vi "函数类型3测试.vi"() -> ()   [LabVIEW 2010]
panel:
  in  "加载配置文件":u16(ring) items=["123.xls", "12333.xls", "1234.xls", "12345.xls", "123666.xls", "12368966.xls"]
  in  "是否取反":bool
  in  "保持输出":bool
  in  "同步_A2":i32
  in  "同步_A1":i32
  in  "数组_输入值":enum16{"0", "1"}[][](array[ring])
  in  "数组_选择?":bool[][](array[boolean])
  in  "btn_置1_5":bool
  in  "btn_置1_4":bool
  in  "btn_置1_3":bool
  in  "btn_置1_2":bool
  in  "btn_全选_5":bool
  in  "btn_全选_4":bool
  in  "btn_全选_3":bool
  in  "btn_全选_2":bool
  in  "btn_置1_1":bool
  in  "btn_全选_1":bool
  in  "CAN端口":u16
  out "light_80":bool
  out "light_79":bool
  out "light_78":bool
  out "light_77":bool
  out "light_76":bool
  out "light_75":bool
  out "light_74":bool
  out "light_73":bool
  out "light_72":bool
  out "light_71":bool
  out "light_70":bool
  out "light_69":bool
  out "light_68":bool
  out "light_67":bool
  out "light_66":bool
  out "light_65":bool
  in  "输入值_73":enum16{"0", "1"}(ring)
  in  "输入值_80":enum16{"0", "1"}(ring)
  in  "输入值_79":enum16{"0", "1"}(ring)
  in  "输入值_78":enum16{"0", "1"}(ring)
  in  "输入值_77":enum16{"0", "1"}(ring)
  in  "输入值_76":enum16{"0", "1"}(ring)
  in  "输入值_75":enum16{"0", "1"}(ring)
  in  "输入值_74":enum16{"0", "1"}(ring)
  in  "输入值_65":enum16{"0", "1"}(ring)
  in  "输入值_72":enum16{"0", "1"}(ring)
  in  "输入值_71":enum16{"0", "1"}(ring)
  in  "输入值_70":enum16{"0", "1"}(ring)
  in  "输入值_69":enum16{"0", "1"}(ring)
  in  "输入值_68":enum16{"0", "1"}(ring)
  in  "输入值_67":enum16{"0", "1"}(ring)
  in  "输入值_66":enum16{"0", "1"}(ring)
  in  "单选_第73路":bool
  in  "单选_第80路":bool
  in  "单选_第79路":bool
  in  "单选_第78路":bool
  in  "单选_第77路":bool
  in  "单选_第76路":bool
  in  "单选_第75路":bool
  in  "单选_第74路":bool
  in  "单选_第65路":bool
  in  "单选_第72路":bool
  in  "单选_第71路":bool
  in  "单选_第70路":bool
  in  "单选_第69路":bool
  in  "单选_第68路":bool
  in  "单选_第67路":bool
  in  "单选_第66路":bool
  out "light_64":bool
  out "light_63":bool
  out "light_62":bool
  out "light_61":bool
  out "light_60":bool
  out "light_59":bool
  out "light_58":bool
  out "light_57":bool
  out "light_56":bool
  out "light_55":bool
  out "light_54":bool
  out "light_53":bool
  out "light_52":bool
  out "light_51":bool
  out "light_50":bool
  out "light_49":bool
  in  "输入值_57":enum16{"0", "1"}(ring)
  in  "输入值_64":enum16{"0", "1"}(ring)
  in  "输入值_63":enum16{"0", "1"}(ring)
  in  "输入值_62":enum16{"0", "1"}(ring)
  in  "输入值_61":enum16{"0", "1"}(ring)
  in  "输入值_60":enum16{"0", "1"}(ring)
  in  "输入值_59":enum16{"0", "1"}(ring)
  in  "输入值_58":enum16{"0", "1"}(ring)
  in  "输入值_49":enum16{"0", "1"}(ring)
  in  "输入值_56":enum16{"0", "1"}(ring)
  in  "输入值_55":enum16{"0", "1"}(ring)
  in  "输入值_54":enum16{"0", "1"}(ring)
  in  "输入值_53":enum16{"0", "1"}(ring)
  in  "输入值_52":enum16{"0", "1"}(ring)
  in  "输入值_51":enum16{"0", "1"}(ring)
  in  "输入值_50":enum16{"0", "1"}(ring)
  in  "单选_第57路":bool
  in  "单选_第64路":bool
  in  "单选_第63路":bool
  in  "单选_第62路":bool
  in  "单选_第61路":bool
  in  "单选_第60路":bool
  in  "单选_第59路":bool
  in  "单选_第58路":bool
  in  "单选_第49路":bool
  in  "单选_第56路":bool
  in  "单选_第55路":bool
  in  "单选_第54路":bool
  in  "单选_第53路":bool
  in  "单选_第52路":bool
  in  "单选_第51路":bool
  in  "单选_第50路":bool
  out "light_48":bool
  out "light_47":bool
  out "light_46":bool
  out "light_45":bool
  out "light_44":bool
  out "light_43":bool
  out "light_42":bool
  out "light_41":bool
  out "light_40":bool
  out "light_39":bool
  out "light_38":bool
  out "light_37":bool
  out "light_36":bool
  out "light_35":bool
  out "light_34":bool
  out "light_33":bool
  in  "输入值_41":enum16{"0", "1"}(ring)
  in  "输入值_48":enum16{"0", "1"}(ring)
  in  "输入值_47":enum16{"0", "1"}(ring)
  in  "输入值_46":enum16{"0", "1"}(ring)
  in  "输入值_45":enum16{"0", "1"}(ring)
  in  "输入值_44":enum16{"0", "1"}(ring)
  in  "输入值_43":enum16{"0", "1"}(ring)
  in  "输入值_42":enum16{"0", "1"}(ring)
  in  "输入值_33":enum16{"0", "1"}(ring)
  in  "输入值_40":enum16{"0", "1"}(ring)
  in  "输入值_39":enum16{"0", "1"}(ring)
  in  "输入值_38":enum16{"0", "1"}(ring)
  in  "输入值_37":enum16{"0", "1"}(ring)
  in  "输入值_36":enum16{"0", "1"}(ring)
  in  "输入值_35":enum16{"0", "1"}(ring)
  in  "输入值_34":enum16{"0", "1"}(ring)
  in  "单选_第41路":bool
  in  "单选_第48路":bool
  in  "单选_第47路":bool
  in  "单选_第46路":bool
  in  "单选_第45路":bool
  in  "单选_第44路":bool
  in  "单选_第43路":bool
  in  "单选_第42路":bool
  in  "单选_第33路":bool
  in  "单选_第40路":bool
  in  "单选_第39路":bool
  in  "单选_第38路":bool
  in  "单选_第37路":bool
  in  "单选_第36路":bool
  in  "单选_第35路":bool
  in  "单选_第34路":bool
  out "light_32":bool
  out "light_31":bool
  out "light_30":bool
  out "light_29":bool
  out "light_28":bool
  out "light_27":bool
  out "light_26":bool
  out "light_25":bool
  out "light_24":bool
  out "light_23":bool
  out "light_22":bool
  out "light_21":bool
  out "light_20":bool
  out "light_19":bool
  out "light_18":bool
  out "light_17":bool
  in  "输入值_25":enum16{"0", "1"}(ring)
  in  "输入值_32":enum16{"0", "1"}(ring)
  in  "输入值_31":enum16{"0", "1"}(ring)
  in  "输入值_30":enum16{"0", "1"}(ring)
  in  "输入值_29":enum16{"0", "1"}(ring)
  in  "输入值_28":enum16{"0", "1"}(ring)
  in  "输入值_27":enum16{"0", "1"}(ring)
  in  "输入值_26":enum16{"0", "1"}(ring)
  in  "输入值_17":enum16{"0", "1"}(ring)
  in  "输入值_24":enum16{"0", "1"}(ring)
  in  "输入值_23":enum16{"0", "1"}(ring)
  in  "输入值_22":enum16{"0", "1"}(ring)
  in  "输入值_21":enum16{"0", "1"}(ring)
  in  "输入值_20":enum16{"0", "1"}(ring)
  in  "输入值_19":enum16{"0", "1"}(ring)
  in  "输入值_18":enum16{"0", "1"}(ring)
  in  "单选_第25路":bool
  in  "单选_第32路":bool
  in  "单选_第31路":bool
  in  "单选_第30路":bool
  in  "单选_第29路":bool
  in  "单选_第28路":bool
  in  "单选_第27路":bool
  in  "单选_第26路":bool
  in  "单选_第17路":bool
  in  "单选_第24路":bool
  in  "单选_第23路":bool
  in  "单选_第22路":bool
  in  "单选_第21路":bool
  in  "单选_第20路":bool
  in  "单选_第19路":bool
  in  "单选_第18路":bool
  in  "D_IN_5":string[][](table) caption="表格"
  in  "D_IN_4":string[][](table) caption="表格"
  in  "D_IN_3":string[][](table) caption="表格"
  in  "D_IN_2":string[][](table) caption="表格"
  out "light_16":bool
  out "light_15":bool
  out "light_14":bool
  out "light_13":bool
  out "light_12":bool
  out "light_11":bool
  out "light_10":bool
  out "light_9":bool
  out "light_8":bool
  out "light_7":bool
  out "light_6":bool
  out "light_5":bool
  out "light_4":bool
  out "light_3":bool
  out "light_2":bool
  out "light_1":bool
  in  "输入值_9":enum16{"0", "1"}(ring)
  in  "输入值_16":enum16{"0", "1"}(ring)
  in  "输入值_15":enum16{"0", "1"}(ring)
  in  "输入值_14":enum16{"0", "1"}(ring)
  in  "输入值_13":enum16{"0", "1"}(ring)
  in  "输入值_12":enum16{"0", "1"}(ring)
  in  "输入值_11":enum16{"0", "1"}(ring)
  in  "输入值_10":enum16{"0", "1"}(ring)
  in  "输入值_1":enum16{"0", "1"}(ring)
  in  "输入值_8":enum16{"0", "1"}(ring)
  in  "输入值_7":enum16{"0", "1"}(ring)
  in  "输入值_6":enum16{"0", "1"}(ring)
  in  "输入值_5":enum16{"0", "1"}(ring)
  in  "输入值_4":enum16{"0", "1"}(ring)
  in  "输入值_3":enum16{"0", "1"}(ring)
  in  "输入值_2":enum16{"0", "1"}(ring)
  in  "单选_第9路":bool
  in  "单选_第16路":bool
  in  "单选_第15路":bool
  in  "单选_第14路":bool
  in  "单选_第13路":bool
  in  "单选_第12路":bool
  in  "单选_第11路":bool
  in  "单选_第10路":bool
  in  "单选_第1路":bool
  in  "单选_第8路":bool
  in  "单选_第7路":bool
  in  "单选_第6路":bool
  in  "单选_第5路":bool
  in  "单选_第4路":bool
  in  "单选_第3路":bool
  in  "单选_第2路":bool
  in  "D_IN_1":string[][](table) caption="表格"
  out "关闭？":bool
  out "测试结论":string
  in  "btn_置0":bool
  in  "btn_置1":bool
  in  "btn_反选":bool
  in  "btn_全选":bool
  in  "btn_关闭":bool
  in  "btn_开始试验":bool
  # "第一组数字量测试"
  # "第二组数字量测试"
  # "第三组数字量测试"
  # "第四组数字量测试"
  # "第五组数字量测试"
  # "加载配置文件："
  # "测试结论："
  # "5X16"
  # "5X16"
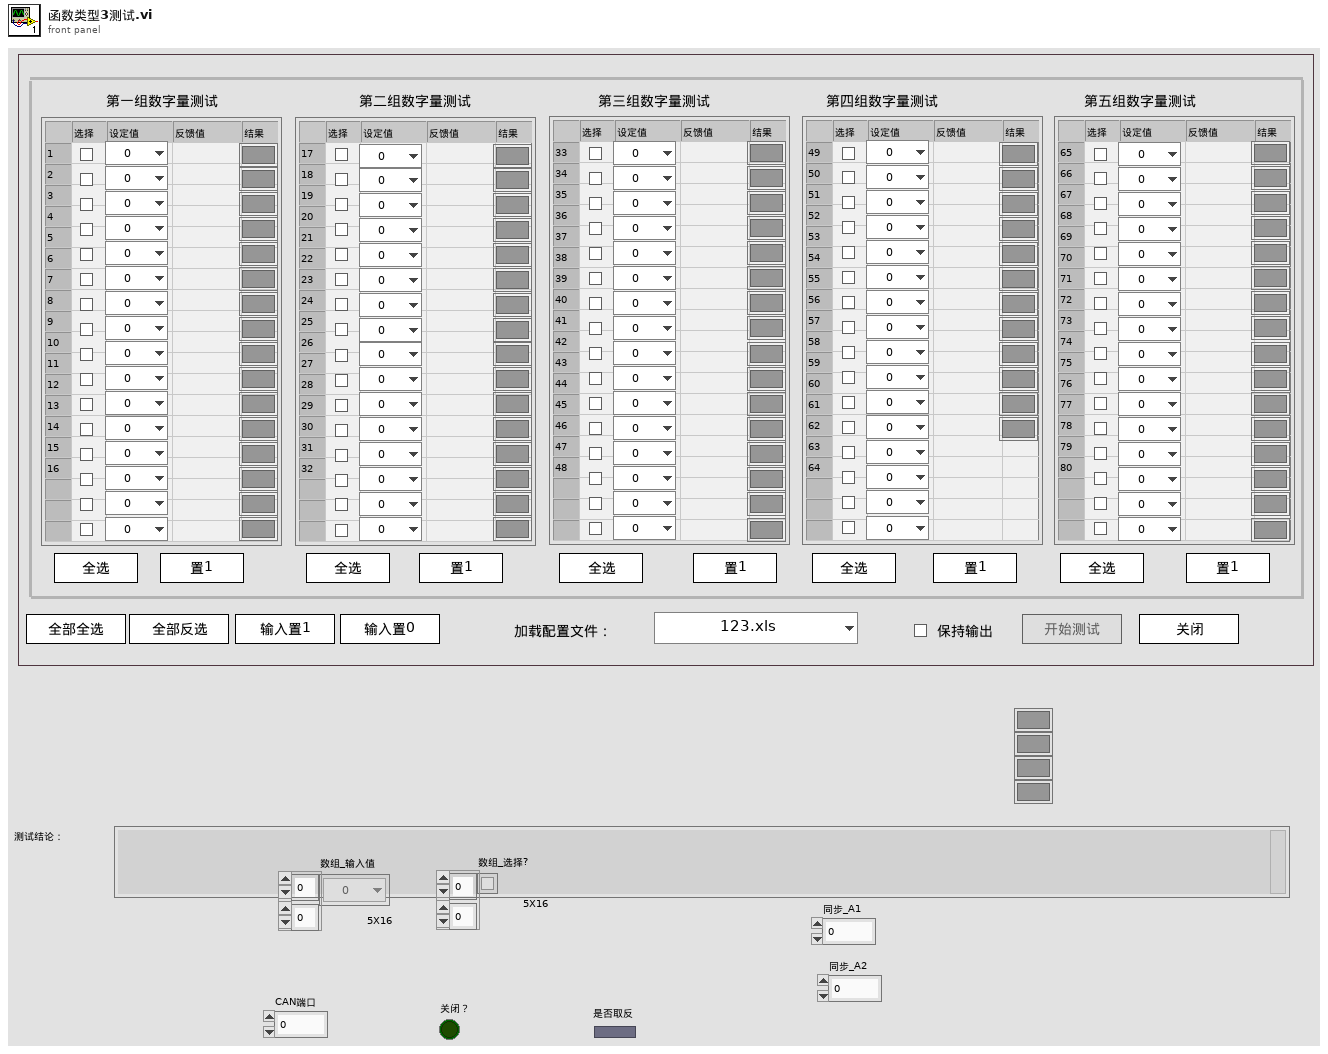
[diagram p1: front panel]
types:
  T1 = enum8{"Enabled", "Disabled", "Disabled and Grayed Out"}
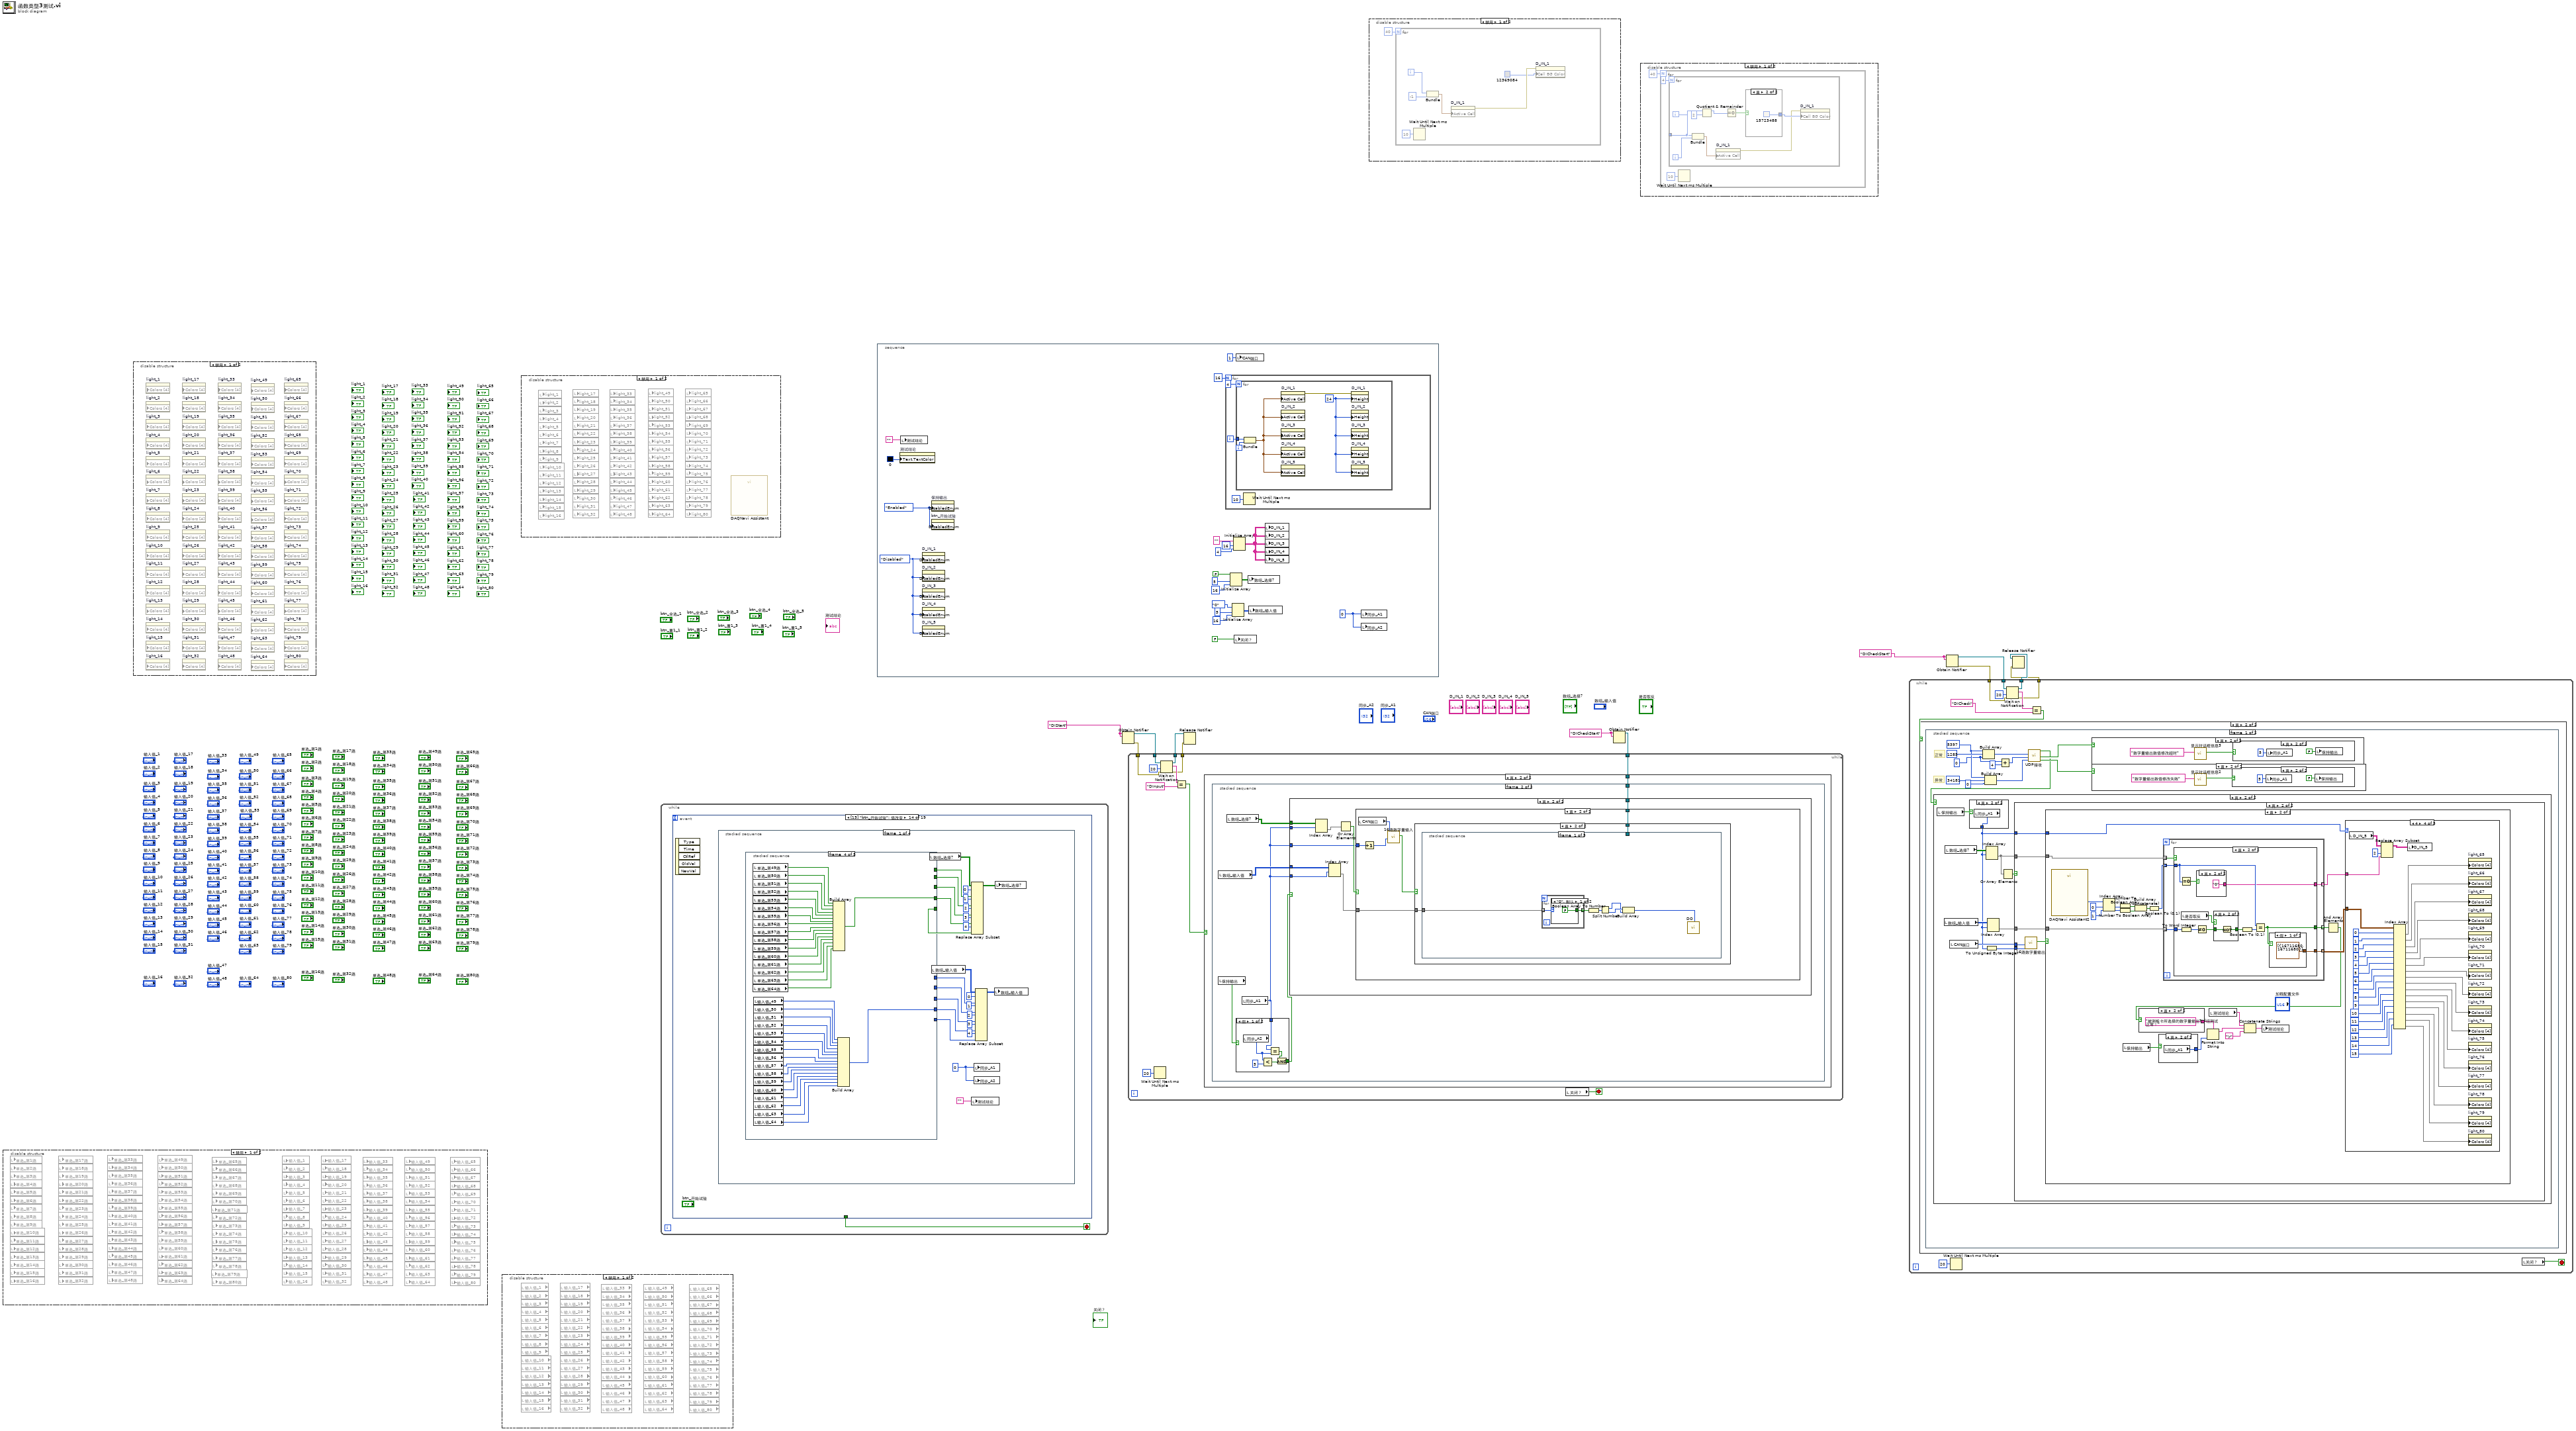
[diagram p0: block diagram]
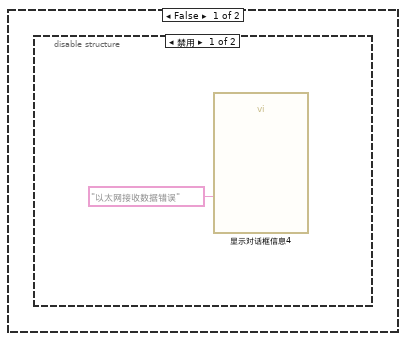
[diagram p7: hidden frame]
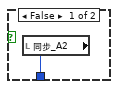
[diagram p9: hidden frame]
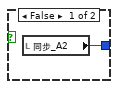
[diagram p12: hidden frame]
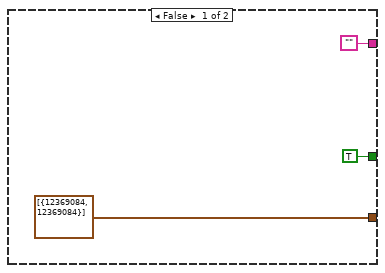
[diagram p13: hidden frame]
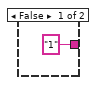
[diagram p15: hidden frame]
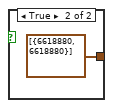
[diagram p16: hidden frame]
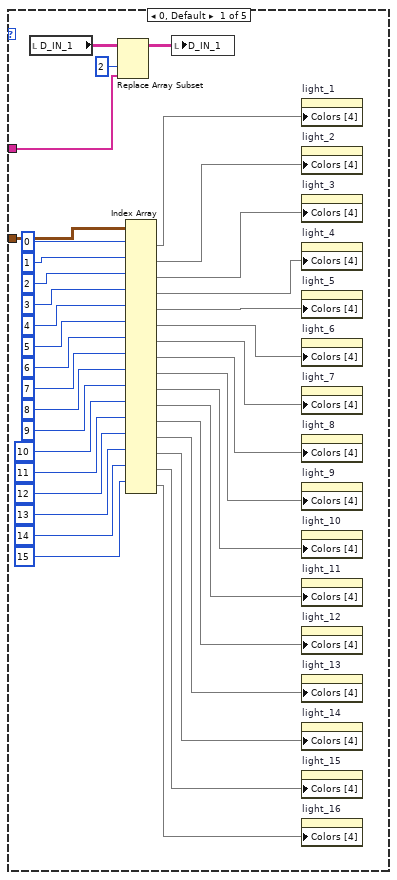
[diagram p17: hidden frame]
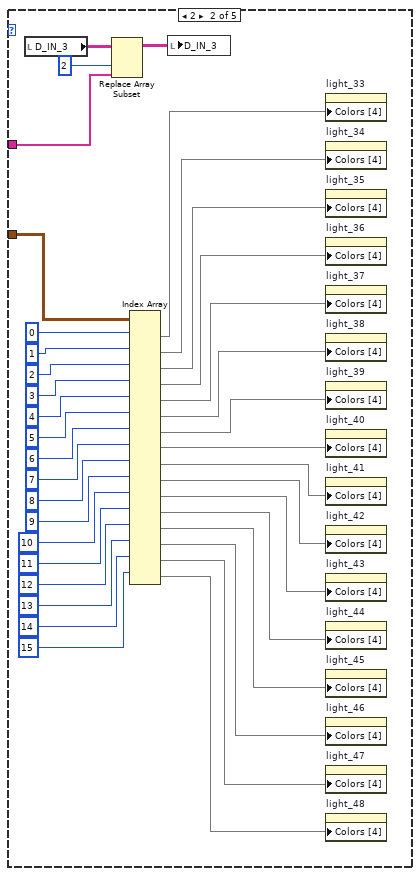
[diagram p18: hidden frame]
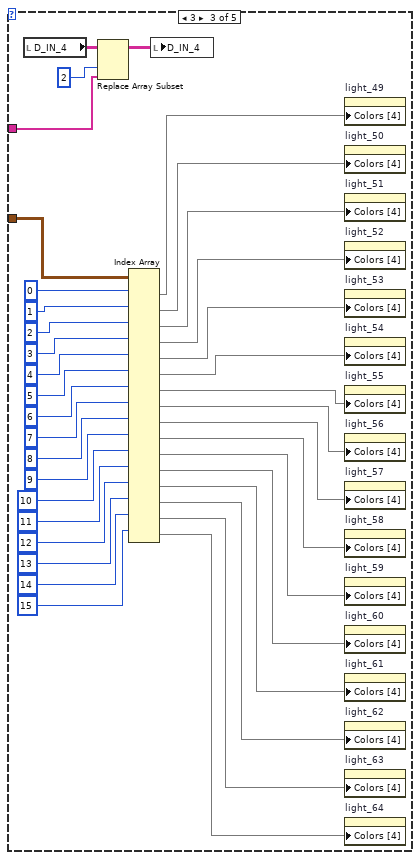
[diagram p19: hidden frame]
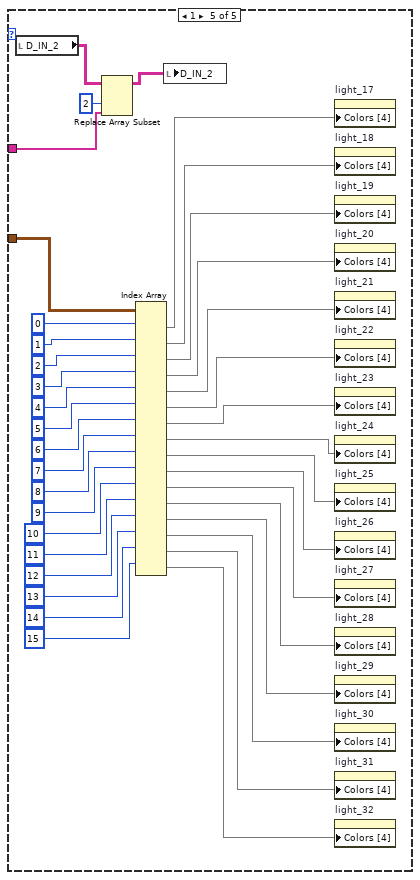
[diagram p20: hidden frame]
diagram:
  w1 = "DICheckStart" ("名称（未命名）")
  w3 = "DICheckStart" ("名称（未命名）")
  w4 = "DIStart" ("名称（未命名）")
  n1 = disable-structure shown="禁用" {
    frame Disabled {
      n2 = local read "单选_第1路"() -> ()  [unwired: 1 in]
      n3 = local read "单选_第2路"() -> ()  [unwired: 1 in]
      n4 = local read "单选_第3路"() -> ()  [unwired: 1 in]
      n5 = local read "单选_第4路"() -> ()  [unwired: 1 in]
      n6 = local read "单选_第5路"() -> ()  [unwired: 1 in]
      n7 = local read "单选_第6路"() -> ()  [unwired: 1 in]
      n8 = local read "单选_第7路"() -> ()  [unwired: 1 in]
      n9 = local read "单选_第8路"() -> ()  [unwired: 1 in]
      n10 = local read "单选_第9路"() -> ()  [unwired: 1 in]
      n11 = local read "单选_第10路"() -> ()  [unwired: 1 in]
      n12 = local read "单选_第11路"() -> ()  [unwired: 1 in]
      n13 = local read "单选_第12路"() -> ()  [unwired: 1 in]
      n14 = local read "单选_第13路"() -> ()  [unwired: 1 in]
      n15 = local read "单选_第14路"() -> ()  [unwired: 1 in]
      n16 = local read "单选_第15路"() -> ()  [unwired: 1 in]
      n17 = local read "单选_第16路"() -> ()  [unwired: 1 in]
      n18 = local read "单选_第17路"() -> ()  [unwired: 1 in]
      n19 = local read "单选_第18路"() -> ()  [unwired: 1 in]
      n20 = local read "单选_第19路"() -> ()  [unwired: 1 in]
      n21 = local read "单选_第20路"() -> ()  [unwired: 1 in]
      n22 = local read "单选_第21路"() -> ()  [unwired: 1 in]
      n23 = local read "单选_第22路"() -> ()  [unwired: 1 in]
      n24 = local read "单选_第23路"() -> ()  [unwired: 1 in]
      n25 = local read "单选_第24路"() -> ()  [unwired: 1 in]
      n26 = local read "单选_第25路"() -> ()  [unwired: 1 in]
      n27 = local read "单选_第26路"() -> ()  [unwired: 1 in]
      n28 = local read "单选_第27路"() -> ()  [unwired: 1 in]
      n29 = local read "单选_第28路"() -> ()  [unwired: 1 in]
      n30 = local read "单选_第29路"() -> ()  [unwired: 1 in]
      n31 = local read "单选_第30路"() -> ()  [unwired: 1 in]
      n32 = local read "单选_第31路"() -> ()  [unwired: 1 in]
      n33 = local read "单选_第32路"() -> ()  [unwired: 1 in]
      n34 = local read "单选_第33路"() -> ()  [unwired: 1 in]
      n35 = local read "单选_第34路"() -> ()  [unwired: 1 in]
      n36 = local read "单选_第35路"() -> ()  [unwired: 1 in]
      n37 = local read "单选_第36路"() -> ()  [unwired: 1 in]
      n38 = local read "单选_第37路"() -> ()  [unwired: 1 in]
      n39 = local read "单选_第38路"() -> ()  [unwired: 1 in]
      n40 = local read "单选_第39路"() -> ()  [unwired: 1 in]
      n41 = local read "单选_第40路"() -> ()  [unwired: 1 in]
      n42 = local read "单选_第41路"() -> ()  [unwired: 1 in]
      n43 = local read "单选_第42路"() -> ()  [unwired: 1 in]
      n44 = local read "单选_第43路"() -> ()  [unwired: 1 in]
      n45 = local read "单选_第44路"() -> ()  [unwired: 1 in]
      n46 = local read "单选_第45路"() -> ()  [unwired: 1 in]
      n47 = local read "单选_第46路"() -> ()  [unwired: 1 in]
      n48 = local read "单选_第47路"() -> ()  [unwired: 1 in]
      n49 = local read "单选_第48路"() -> ()  [unwired: 1 in]
      n50 = local read "单选_第49路"() -> ()  [unwired: 1 in]
      n51 = local read "单选_第50路"() -> ()  [unwired: 1 in]
      n52 = local read "单选_第51路"() -> ()  [unwired: 1 in]
      n53 = local read "单选_第52路"() -> ()  [unwired: 1 in]
      n54 = local read "单选_第53路"() -> ()  [unwired: 1 in]
      n55 = local read "单选_第54路"() -> ()  [unwired: 1 in]
      n56 = local read "单选_第55路"() -> ()  [unwired: 1 in]
      n57 = local read "单选_第56路"() -> ()  [unwired: 1 in]
      n58 = local read "单选_第57路"() -> ()  [unwired: 1 in]
      n59 = local read "单选_第58路"() -> ()  [unwired: 1 in]
      n60 = local read "单选_第59路"() -> ()  [unwired: 1 in]
      n61 = local read "单选_第60路"() -> ()  [unwired: 1 in]
      n62 = local read "单选_第61路"() -> ()  [unwired: 1 in]
      n63 = local read "单选_第62路"() -> ()  [unwired: 1 in]
      n64 = local read "单选_第63路"() -> ()  [unwired: 1 in]
      n65 = local read "单选_第64路"() -> ()  [unwired: 1 in]
      n66 = local read "单选_第71路"() -> ()  [unwired: 1 in]
      n67 = local read "单选_第79路"() -> ()  [unwired: 1 in]
      n68 = local read "单选_第65路"() -> ()  [unwired: 1 in]
      n69 = local read "单选_第66路"() -> ()  [unwired: 1 in]
      n70 = local read "单选_第67路"() -> ()  [unwired: 1 in]
      n71 = local read "单选_第68路"() -> ()  [unwired: 1 in]
      n72 = local read "单选_第69路"() -> ()  [unwired: 1 in]
      n73 = local read "单选_第70路"() -> ()  [unwired: 1 in]
      n74 = local read "单选_第72路"() -> ()  [unwired: 1 in]
      n75 = local read "单选_第73路"() -> ()  [unwired: 1 in]
      n76 = local read "单选_第74路"() -> ()  [unwired: 1 in]
      n77 = local read "单选_第75路"() -> ()  [unwired: 1 in]
      n78 = local read "单选_第76路"() -> ()  [unwired: 1 in]
      n79 = local read "单选_第77路"() -> ()  [unwired: 1 in]
      n80 = local read "单选_第78路"() -> ()  [unwired: 1 in]
      n81 = local read "单选_第80路"() -> ()  [unwired: 1 in]
      n82 = local read "输入值_1"() -> ()  [unwired: 1 in]
      n83 = local read "输入值_2"() -> ()  [unwired: 1 in]
      n84 = local read "输入值_3"() -> ()  [unwired: 1 in]
      n85 = local read "输入值_4"() -> ()  [unwired: 1 in]
      n86 = local read "输入值_5"() -> ()  [unwired: 1 in]
      n87 = local read "输入值_6"() -> ()  [unwired: 1 in]
      n88 = local read "输入值_7"() -> ()  [unwired: 1 in]
      n89 = local read "输入值_8"() -> ()  [unwired: 1 in]
      n90 = local read "输入值_9"() -> ()  [unwired: 1 in]
      n91 = local read "输入值_10"() -> ()  [unwired: 1 in]
      n92 = local read "输入值_11"() -> ()  [unwired: 1 in]
      n93 = local read "输入值_12"() -> ()  [unwired: 1 in]
      n94 = local read "输入值_13"() -> ()  [unwired: 1 in]
      n95 = local read "输入值_14"() -> ()  [unwired: 1 in]
      n96 = local read "输入值_15"() -> ()  [unwired: 1 in]
      n97 = local read "输入值_16"() -> ()  [unwired: 1 in]
      n98 = local read "输入值_17"() -> ()  [unwired: 1 in]
      n99 = local read "输入值_18"() -> ()  [unwired: 1 in]
      n100 = local read "输入值_19"() -> ()  [unwired: 1 in]
      n101 = local read "输入值_20"() -> ()  [unwired: 1 in]
      n102 = local read "输入值_21"() -> ()  [unwired: 1 in]
      n103 = local read "输入值_22"() -> ()  [unwired: 1 in]
      n104 = local read "输入值_23"() -> ()  [unwired: 1 in]
      n105 = local read "输入值_24"() -> ()  [unwired: 1 in]
      n106 = local read "输入值_25"() -> ()  [unwired: 1 in]
      n107 = local read "输入值_26"() -> ()  [unwired: 1 in]
      n108 = local read "输入值_27"() -> ()  [unwired: 1 in]
      n109 = local read "输入值_28"() -> ()  [unwired: 1 in]
      n110 = local read "输入值_29"() -> ()  [unwired: 1 in]
      n111 = local read "输入值_30"() -> ()  [unwired: 1 in]
      n112 = local read "输入值_31"() -> ()  [unwired: 1 in]
      n113 = local read "输入值_32"() -> ()  [unwired: 1 in]
      n114 = local read "输入值_33"() -> ()  [unwired: 1 in]
      n115 = local read "输入值_34"() -> ()  [unwired: 1 in]
      n116 = local read "输入值_35"() -> ()  [unwired: 1 in]
      n117 = local read "输入值_36"() -> ()  [unwired: 1 in]
      n118 = local read "输入值_37"() -> ()  [unwired: 1 in]
      n119 = local read "输入值_38"() -> ()  [unwired: 1 in]
      n120 = local read "输入值_39"() -> ()  [unwired: 1 in]
      n121 = local read "输入值_40"() -> ()  [unwired: 1 in]
      n122 = local read "输入值_41"() -> ()  [unwired: 1 in]
      n123 = local read "输入值_42"() -> ()  [unwired: 1 in]
      n124 = local read "输入值_43"() -> ()  [unwired: 1 in]
      n125 = local read "输入值_44"() -> ()  [unwired: 1 in]
      n126 = local read "输入值_45"() -> ()  [unwired: 1 in]
      n127 = local read "输入值_46"() -> ()  [unwired: 1 in]
      n128 = local read "输入值_47"() -> ()  [unwired: 1 in]
      n129 = local read "输入值_48"() -> ()  [unwired: 1 in]
      n130 = local read "输入值_49"() -> ()  [unwired: 1 in]
      n131 = local read "输入值_50"() -> ()  [unwired: 1 in]
      n132 = local read "输入值_51"() -> ()  [unwired: 1 in]
      n133 = local read "输入值_52"() -> ()  [unwired: 1 in]
      n134 = local read "输入值_53"() -> ()  [unwired: 1 in]
      n135 = local read "输入值_54"() -> ()  [unwired: 1 in]
      n136 = local read "输入值_55"() -> ()  [unwired: 1 in]
      n137 = local read "输入值_56"() -> ()  [unwired: 1 in]
      n138 = local read "输入值_57"() -> ()  [unwired: 1 in]
      n139 = local read "输入值_58"() -> ()  [unwired: 1 in]
      n140 = local read "输入值_59"() -> ()  [unwired: 1 in]
      n141 = local read "输入值_60"() -> ()  [unwired: 1 in]
      n142 = local read "输入值_61"() -> ()  [unwired: 1 in]
      n143 = local read "输入值_62"() -> ()  [unwired: 1 in]
      n144 = local read "输入值_63"() -> ()  [unwired: 1 in]
      n145 = local read "输入值_64"() -> ()  [unwired: 1 in]
      n146 = local read "输入值_65"() -> ()  [unwired: 1 in]
      n147 = local read "输入值_66"() -> ()  [unwired: 1 in]
      n148 = local read "输入值_67"() -> ()  [unwired: 1 in]
      n149 = local read "输入值_68"() -> ()  [unwired: 1 in]
      n150 = local read "输入值_69"() -> ()  [unwired: 1 in]
      n151 = local read "输入值_70"() -> ()  [unwired: 1 in]
      n152 = local read "输入值_71"() -> ()  [unwired: 1 in]
      n153 = local read "输入值_72"() -> ()  [unwired: 1 in]
      n154 = local read "输入值_73"() -> ()  [unwired: 1 in]
      n155 = local read "输入值_74"() -> ()  [unwired: 1 in]
      n156 = local read "输入值_75"() -> ()  [unwired: 1 in]
      n157 = local read "输入值_76"() -> ()  [unwired: 1 in]
      n158 = local read "输入值_77"() -> ()  [unwired: 1 in]
      n159 = local read "输入值_78"() -> ()  [unwired: 1 in]
      n160 = local read "输入值_79"() -> ()  [unwired: 1 in]
      n161 = local read "输入值_80"() -> ()  [unwired: 1 in]
    }
    frame Enabled {
    }
  }
  n162 = disable-structure shown="禁用" {
    frame Disabled {
      n163 = property on="light_1" class="Bool (严格)" props=["Colors [4]"]() -> ()  [unwired: 3 in, 2 out]
      n164 = property on="light_2" class="Bool (严格)" props=["Colors [4]"]() -> ()  [unwired: 3 in, 2 out]
      n165 = property on="light_3" class="Bool (严格)" props=["Colors [4]"]() -> ()  [unwired: 3 in, 2 out]
      n166 = property on="light_4" class="Bool (严格)" props=["Colors [4]"]() -> ()  [unwired: 3 in, 2 out]
      n167 = property on="light_5" class="Bool (严格)" props=["Colors [4]"]() -> ()  [unwired: 3 in, 2 out]
      n168 = property on="light_6" class="Bool (严格)" props=["Colors [4]"]() -> ()  [unwired: 3 in, 2 out]
      n169 = property on="light_7" class="Bool (严格)" props=["Colors [4]"]() -> ()  [unwired: 3 in, 2 out]
      n170 = property on="light_8" class="Bool (严格)" props=["Colors [4]"]() -> ()  [unwired: 3 in, 2 out]
      n171 = property on="light_9" class="Bool (严格)" props=["Colors [4]"]() -> ()  [unwired: 3 in, 2 out]
      n172 = property on="light_10" class="Bool (严格)" props=["Colors [4]"]() -> ()  [unwired: 3 in, 2 out]
      n173 = property on="light_11" class="Bool (严格)" props=["Colors [4]"]() -> ()  [unwired: 3 in, 2 out]
      n174 = property on="light_12" class="Bool (严格)" props=["Colors [4]"]() -> ()  [unwired: 3 in, 2 out]
      n175 = property on="light_13" class="Bool (严格)" props=["Colors [4]"]() -> ()  [unwired: 3 in, 2 out]
      n176 = property on="light_14" class="Bool (严格)" props=["Colors [4]"]() -> ()  [unwired: 3 in, 2 out]
      n177 = property on="light_15" class="Bool (严格)" props=["Colors [4]"]() -> ()  [unwired: 3 in, 2 out]
      n178 = property on="light_16" class="Bool (严格)" props=["Colors [4]"]() -> ()  [unwired: 3 in, 2 out]
      n179 = property on="light_17" class="Bool (严格)" props=["Colors [4]"]() -> ()  [unwired: 3 in, 2 out]
      n180 = property on="light_18" class="Bool (严格)" props=["Colors [4]"]() -> ()  [unwired: 3 in, 2 out]
      n181 = property on="light_19" class="Bool (严格)" props=["Colors [4]"]() -> ()  [unwired: 3 in, 2 out]
      n182 = property on="light_20" class="Bool (严格)" props=["Colors [4]"]() -> ()  [unwired: 3 in, 2 out]
      n183 = property on="light_21" class="Bool (严格)" props=["Colors [4]"]() -> ()  [unwired: 3 in, 2 out]
      n184 = property on="light_22" class="Bool (严格)" props=["Colors [4]"]() -> ()  [unwired: 3 in, 2 out]
      n185 = property on="light_23" class="Bool (严格)" props=["Colors [4]"]() -> ()  [unwired: 3 in, 2 out]
      n186 = property on="light_24" class="Bool (严格)" props=["Colors [4]"]() -> ()  [unwired: 3 in, 2 out]
      n187 = property on="light_25" class="Bool (严格)" props=["Colors [4]"]() -> ()  [unwired: 3 in, 2 out]
      n188 = property on="light_26" class="Bool (严格)" props=["Colors [4]"]() -> ()  [unwired: 3 in, 2 out]
      n189 = property on="light_27" class="Bool (严格)" props=["Colors [4]"]() -> ()  [unwired: 3 in, 2 out]
      n190 = property on="light_28" class="Bool (严格)" props=["Colors [4]"]() -> ()  [unwired: 3 in, 2 out]
      n191 = property on="light_29" class="Bool (严格)" props=["Colors [4]"]() -> ()  [unwired: 3 in, 2 out]
      n192 = property on="light_30" class="Bool (严格)" props=["Colors [4]"]() -> ()  [unwired: 3 in, 2 out]
      n193 = property on="light_31" class="Bool (严格)" props=["Colors [4]"]() -> ()  [unwired: 3 in, 2 out]
      n194 = property on="light_32" class="Bool (严格)" props=["Colors [4]"]() -> ()  [unwired: 3 in, 2 out]
      n195 = property on="light_33" class="Bool (严格)" props=["Colors [4]"]() -> ()  [unwired: 3 in, 2 out]
      n196 = property on="light_34" class="Bool (严格)" props=["Colors [4]"]() -> ()  [unwired: 3 in, 2 out]
      n197 = property on="light_35" class="Bool (严格)" props=["Colors [4]"]() -> ()  [unwired: 3 in, 2 out]
      n198 = property on="light_36" class="Bool (严格)" props=["Colors [4]"]() -> ()  [unwired: 3 in, 2 out]
      n199 = property on="light_37" class="Bool (严格)" props=["Colors [4]"]() -> ()  [unwired: 3 in, 2 out]
      n200 = property on="light_38" class="Bool (严格)" props=["Colors [4]"]() -> ()  [unwired: 3 in, 2 out]
      n201 = property on="light_39" class="Bool (严格)" props=["Colors [4]"]() -> ()  [unwired: 3 in, 2 out]
      n202 = property on="light_40" class="Bool (严格)" props=["Colors [4]"]() -> ()  [unwired: 3 in, 2 out]
      n203 = property on="light_41" class="Bool (严格)" props=["Colors [4]"]() -> ()  [unwired: 3 in, 2 out]
      n204 = property on="light_42" class="Bool (严格)" props=["Colors [4]"]() -> ()  [unwired: 3 in, 2 out]
      n205 = property on="light_43" class="Bool (严格)" props=["Colors [4]"]() -> ()  [unwired: 3 in, 2 out]
      n206 = property on="light_44" class="Bool (严格)" props=["Colors [4]"]() -> ()  [unwired: 3 in, 2 out]
      n207 = property on="light_45" class="Bool (严格)" props=["Colors [4]"]() -> ()  [unwired: 3 in, 2 out]
      n208 = property on="light_46" class="Bool (严格)" props=["Colors [4]"]() -> ()  [unwired: 3 in, 2 out]
      n209 = property on="light_47" class="Bool (严格)" props=["Colors [4]"]() -> ()  [unwired: 3 in, 2 out]
      n210 = property on="light_48" class="Bool (严格)" props=["Colors [4]"]() -> ()  [unwired: 3 in, 2 out]
      n211 = property on="light_49" class="Bool (严格)" props=["Colors [4]"]() -> ()  [unwired: 3 in, 2 out]
      n212 = property on="light_50" class="Bool (严格)" props=["Colors [4]"]() -> ()  [unwired: 3 in, 2 out]
      n213 = property on="light_51" class="Bool (严格)" props=["Colors [4]"]() -> ()  [unwired: 3 in, 2 out]
      n214 = property on="light_52" class="Bool (严格)" props=["Colors [4]"]() -> ()  [unwired: 3 in, 2 out]
      n215 = property on="light_53" class="Bool (严格)" props=["Colors [4]"]() -> ()  [unwired: 3 in, 2 out]
      n216 = property on="light_54" class="Bool (严格)" props=["Colors [4]"]() -> ()  [unwired: 3 in, 2 out]
      n217 = property on="light_55" class="Bool (严格)" props=["Colors [4]"]() -> ()  [unwired: 3 in, 2 out]
      n218 = property on="light_56" class="Bool (严格)" props=["Colors [4]"]() -> ()  [unwired: 3 in, 2 out]
      n219 = property on="light_57" class="Bool (严格)" props=["Colors [4]"]() -> ()  [unwired: 3 in, 2 out]
      n220 = property on="light_58" class="Bool (严格)" props=["Colors [4]"]() -> ()  [unwired: 3 in, 2 out]
      n221 = property on="light_59" class="Bool (严格)" props=["Colors [4]"]() -> ()  [unwired: 3 in, 2 out]
      n222 = property on="light_60" class="Bool (严格)" props=["Colors [4]"]() -> ()  [unwired: 3 in, 2 out]
      n223 = property on="light_61" class="Bool (严格)" props=["Colors [4]"]() -> ()  [unwired: 3 in, 2 out]
      n224 = property on="light_62" class="Bool (严格)" props=["Colors [4]"]() -> ()  [unwired: 3 in, 2 out]
      n225 = property on="light_63" class="Bool (严格)" props=["Colors [4]"]() -> ()  [unwired: 3 in, 2 out]
      n226 = property on="light_64" class="Bool (严格)" props=["Colors [4]"]() -> ()  [unwired: 3 in, 2 out]
      n227 = property on="light_65" class="Bool (严格)" props=["Colors [4]"]() -> ()  [unwired: 3 in, 2 out]
      n228 = property on="light_66" class="Bool (严格)" props=["Colors [4]"]() -> ()  [unwired: 3 in, 2 out]
      n229 = property on="light_67" class="Bool (严格)" props=["Colors [4]"]() -> ()  [unwired: 3 in, 2 out]
      n230 = property on="light_68" class="Bool (严格)" props=["Colors [4]"]() -> ()  [unwired: 3 in, 2 out]
      n231 = property on="light_69" class="Bool (严格)" props=["Colors [4]"]() -> ()  [unwired: 3 in, 2 out]
      n232 = property on="light_70" class="Bool (严格)" props=["Colors [4]"]() -> ()  [unwired: 3 in, 2 out]
      n233 = property on="light_71" class="Bool (严格)" props=["Colors [4]"]() -> ()  [unwired: 3 in, 2 out]
      n234 = property on="light_72" class="Bool (严格)" props=["Colors [4]"]() -> ()  [unwired: 3 in, 2 out]
      n235 = property on="light_73" class="Bool (严格)" props=["Colors [4]"]() -> ()  [unwired: 3 in, 2 out]
      n236 = property on="light_74" class="Bool (严格)" props=["Colors [4]"]() -> ()  [unwired: 3 in, 2 out]
      n237 = property on="light_75" class="Bool (严格)" props=["Colors [4]"]() -> ()  [unwired: 3 in, 2 out]
      n238 = property on="light_76" class="Bool (严格)" props=["Colors [4]"]() -> ()  [unwired: 3 in, 2 out]
      n239 = property on="light_77" class="Bool (严格)" props=["Colors [4]"]() -> ()  [unwired: 3 in, 2 out]
      n240 = property on="light_78" class="Bool (严格)" props=["Colors [4]"]() -> ()  [unwired: 3 in, 2 out]
      n241 = property on="light_79" class="Bool (严格)" props=["Colors [4]"]() -> ()  [unwired: 3 in, 2 out]
      n242 = property on="light_80" class="Bool (严格)" props=["Colors [4]"]() -> ()  [unwired: 3 in, 2 out]
    }
    frame Enabled {
    }
  }
  n243 = disable-structure shown="禁用" {
    frame Disabled {
      n244 = local read "输入值_1"() -> ()  [unwired: 1 out]
      n245 = local read "输入值_2"() -> ()  [unwired: 1 out]
      n246 = local read "输入值_3"() -> ()  [unwired: 1 out]
      n247 = local read "输入值_4"() -> ()  [unwired: 1 out]
      n248 = local read "输入值_5"() -> ()  [unwired: 1 out]
      n249 = local read "输入值_6"() -> ()  [unwired: 1 out]
      n250 = local read "输入值_7"() -> ()  [unwired: 1 out]
      n251 = local read "输入值_8"() -> ()  [unwired: 1 out]
      n252 = local read "输入值_9"() -> ()  [unwired: 1 out]
      n253 = local read "输入值_10"() -> ()  [unwired: 1 out]
      n254 = local read "输入值_11"() -> ()  [unwired: 1 out]
      n255 = local read "输入值_12"() -> ()  [unwired: 1 out]
      n256 = local read "输入值_13"() -> ()  [unwired: 1 out]
      n257 = local read "输入值_14"() -> ()  [unwired: 1 out]
      n258 = local read "输入值_15"() -> ()  [unwired: 1 out]
      n259 = local read "输入值_16"() -> ()  [unwired: 1 out]
      n260 = local read "输入值_17"() -> ()  [unwired: 1 out]
      n261 = local read "输入值_18"() -> ()  [unwired: 1 out]
      n262 = local read "输入值_19"() -> ()  [unwired: 1 out]
      n263 = local read "输入值_20"() -> ()  [unwired: 1 out]
      n264 = local read "输入值_21"() -> ()  [unwired: 1 out]
      n265 = local read "输入值_22"() -> ()  [unwired: 1 out]
      n266 = local read "输入值_23"() -> ()  [unwired: 1 out]
      n267 = local read "输入值_24"() -> ()  [unwired: 1 out]
      n268 = local read "输入值_25"() -> ()  [unwired: 1 out]
      n269 = local read "输入值_26"() -> ()  [unwired: 1 out]
      n270 = local read "输入值_27"() -> ()  [unwired: 1 out]
      n271 = local read "输入值_28"() -> ()  [unwired: 1 out]
      n272 = local read "输入值_29"() -> ()  [unwired: 1 out]
      n273 = local read "输入值_30"() -> ()  [unwired: 1 out]
      n274 = local read "输入值_31"() -> ()  [unwired: 1 out]
      n275 = local read "输入值_32"() -> ()  [unwired: 1 out]
      n276 = local read "输入值_33"() -> ()  [unwired: 1 out]
      n277 = local read "输入值_34"() -> ()  [unwired: 1 out]
      n278 = local read "输入值_35"() -> ()  [unwired: 1 out]
      n279 = local read "输入值_36"() -> ()  [unwired: 1 out]
      n280 = local read "输入值_37"() -> ()  [unwired: 1 out]
      n281 = local read "输入值_38"() -> ()  [unwired: 1 out]
      n282 = local read "输入值_39"() -> ()  [unwired: 1 out]
      n283 = local read "输入值_40"() -> ()  [unwired: 1 out]
      n284 = local read "输入值_41"() -> ()  [unwired: 1 out]
      n285 = local read "输入值_42"() -> ()  [unwired: 1 out]
      n286 = local read "输入值_43"() -> ()  [unwired: 1 out]
      n287 = local read "输入值_44"() -> ()  [unwired: 1 out]
      n288 = local read "输入值_45"() -> ()  [unwired: 1 out]
      n289 = local read "输入值_46"() -> ()  [unwired: 1 out]
      n290 = local read "输入值_47"() -> ()  [unwired: 1 out]
      n291 = local read "输入值_48"() -> ()  [unwired: 1 out]
      n292 = local read "输入值_49"() -> ()  [unwired: 1 out]
      n293 = local read "输入值_50"() -> ()  [unwired: 1 out]
      n294 = local read "输入值_51"() -> ()  [unwired: 1 out]
      n295 = local read "输入值_52"() -> ()  [unwired: 1 out]
      n296 = local read "输入值_53"() -> ()  [unwired: 1 out]
      n297 = local read "输入值_54"() -> ()  [unwired: 1 out]
      n298 = local read "输入值_55"() -> ()  [unwired: 1 out]
      n299 = local read "输入值_56"() -> ()  [unwired: 1 out]
      n300 = local read "输入值_57"() -> ()  [unwired: 1 out]
      n301 = local read "输入值_58"() -> ()  [unwired: 1 out]
      n302 = local read "输入值_59"() -> ()  [unwired: 1 out]
      n303 = local read "输入值_60"() -> ()  [unwired: 1 out]
      n304 = local read "输入值_61"() -> ()  [unwired: 1 out]
      n305 = local read "输入值_62"() -> ()  [unwired: 1 out]
      n306 = local read "输入值_63"() -> ()  [unwired: 1 out]
      n307 = local read "输入值_64"() -> ()  [unwired: 1 out]
      n308 = local read "输入值_65"() -> ()  [unwired: 1 out]
      n309 = local read "输入值_66"() -> ()  [unwired: 1 out]
      n310 = local read "输入值_67"() -> ()  [unwired: 1 out]
      n311 = local read "输入值_68"() -> ()  [unwired: 1 out]
      n312 = local read "输入值_69"() -> ()  [unwired: 1 out]
      n313 = local read "输入值_70"() -> ()  [unwired: 1 out]
      n314 = local read "输入值_71"() -> ()  [unwired: 1 out]
      n315 = local read "输入值_72"() -> ()  [unwired: 1 out]
      n316 = local read "输入值_73"() -> ()  [unwired: 1 out]
      n317 = local read "输入值_74"() -> ()  [unwired: 1 out]
      n318 = local read "输入值_75"() -> ()  [unwired: 1 out]
      n319 = local read "输入值_76"() -> ()  [unwired: 1 out]
      n320 = local read "输入值_77"() -> ()  [unwired: 1 out]
      n321 = local read "输入值_78"() -> ()  [unwired: 1 out]
      n322 = local read "输入值_79"() -> ()  [unwired: 1 out]
      n323 = local read "输入值_80"() -> ()  [unwired: 1 out]
    }
    frame Enabled {
    }
  }
  n324 = disable-structure shown="禁用" {
    frame Disabled {
      n325 = local read "light_1"() -> ()  [unwired: 1 in]
      n326 = local read "light_2"() -> ()  [unwired: 1 in]
      n327 = local read "light_3"() -> ()  [unwired: 1 in]
      n328 = local read "light_4"() -> ()  [unwired: 1 in]
      n329 = local read "light_5"() -> ()  [unwired: 1 in]
      n330 = local read "light_6"() -> ()  [unwired: 1 in]
      n331 = local read "light_7"() -> ()  [unwired: 1 in]
      n332 = local read "light_8"() -> ()  [unwired: 1 in]
      n333 = local read "light_9"() -> ()  [unwired: 1 in]
      n334 = local read "light_10"() -> ()  [unwired: 1 in]
      n335 = local read "light_11"() -> ()  [unwired: 1 in]
      n336 = local read "light_12"() -> ()  [unwired: 1 in]
      n337 = local read "light_13"() -> ()  [unwired: 1 in]
      n338 = local read "light_14"() -> ()  [unwired: 1 in]
      n339 = local read "light_15"() -> ()  [unwired: 1 in]
      n340 = local read "light_16"() -> ()  [unwired: 1 in]
      n341 = local read "light_17"() -> ()  [unwired: 1 in]
      n342 = local read "light_18"() -> ()  [unwired: 1 in]
      n343 = local read "light_19"() -> ()  [unwired: 1 in]
      n344 = local read "light_20"() -> ()  [unwired: 1 in]
      n345 = local read "light_21"() -> ()  [unwired: 1 in]
      n346 = local read "light_22"() -> ()  [unwired: 1 in]
      n347 = local read "light_23"() -> ()  [unwired: 1 in]
      n348 = local read "light_24"() -> ()  [unwired: 1 in]
      n349 = local read "light_25"() -> ()  [unwired: 1 in]
      n350 = local read "light_26"() -> ()  [unwired: 1 in]
      n351 = local read "light_27"() -> ()  [unwired: 1 in]
      n352 = local read "light_28"() -> ()  [unwired: 1 in]
      n353 = local read "light_29"() -> ()  [unwired: 1 in]
      n354 = local read "light_30"() -> ()  [unwired: 1 in]
      n355 = local read "light_31"() -> ()  [unwired: 1 in]
      n356 = local read "light_32"() -> ()  [unwired: 1 in]
      n357 = local read "light_33"() -> ()  [unwired: 1 in]
      n358 = local read "light_34"() -> ()  [unwired: 1 in]
      n359 = local read "light_35"() -> ()  [unwired: 1 in]
      n360 = local read "light_36"() -> ()  [unwired: 1 in]
      n361 = local read "light_37"() -> ()  [unwired: 1 in]
      n362 = local read "light_38"() -> ()  [unwired: 1 in]
      n363 = local read "light_39"() -> ()  [unwired: 1 in]
      n364 = local read "light_40"() -> ()  [unwired: 1 in]
      n365 = local read "light_41"() -> ()  [unwired: 1 in]
      n366 = local read "light_42"() -> ()  [unwired: 1 in]
      n367 = local read "light_43"() -> ()  [unwired: 1 in]
      n368 = local read "light_44"() -> ()  [unwired: 1 in]
      n369 = local read "light_45"() -> ()  [unwired: 1 in]
      n370 = local read "light_46"() -> ()  [unwired: 1 in]
      n371 = local read "light_47"() -> ()  [unwired: 1 in]
      n372 = local read "light_48"() -> ()  [unwired: 1 in]
      n373 = local read "light_49"() -> ()  [unwired: 1 in]
      n374 = local read "light_50"() -> ()  [unwired: 1 in]
      n375 = local read "light_51"() -> ()  [unwired: 1 in]
      n376 = local read "light_52"() -> ()  [unwired: 1 in]
      n377 = local read "light_53"() -> ()  [unwired: 1 in]
      n378 = local read "light_54"() -> ()  [unwired: 1 in]
      n379 = local read "light_55"() -> ()  [unwired: 1 in]
      n380 = local read "light_56"() -> ()  [unwired: 1 in]
      n381 = local read "light_57"() -> ()  [unwired: 1 in]
      n382 = local read "light_58"() -> ()  [unwired: 1 in]
      n383 = local read "light_59"() -> ()  [unwired: 1 in]
      n384 = local read "light_60"() -> ()  [unwired: 1 in]
      n385 = local read "light_61"() -> ()  [unwired: 1 in]
      n386 = local read "light_62"() -> ()  [unwired: 1 in]
      n387 = local read "light_63"() -> ()  [unwired: 1 in]
      n388 = local read "light_64"() -> ()  [unwired: 1 in]
      n389 = local read "light_65"() -> ()  [unwired: 1 in]
      n390 = local read "light_66"() -> ()  [unwired: 1 in]
      n391 = local read "light_67"() -> ()  [unwired: 1 in]
      n392 = local read "light_68"() -> ()  [unwired: 1 in]
      n393 = local read "light_69"() -> ()  [unwired: 1 in]
      n394 = local read "light_70"() -> ()  [unwired: 1 in]
      n395 = local read "light_71"() -> ()  [unwired: 1 in]
      n396 = local read "light_72"() -> ()  [unwired: 1 in]
      n397 = local read "light_73"() -> ()  [unwired: 1 in]
      n398 = local read "light_74"() -> ()  [unwired: 1 in]
      n399 = local read "light_75"() -> ()  [unwired: 1 in]
      n400 = local read "light_76"() -> ()  [unwired: 1 in]
      n401 = local read "light_77"() -> ()  [unwired: 1 in]
      n402 = local read "light_78"() -> ()  [unwired: 1 in]
      n403 = local read "light_79"() -> ()  [unwired: 1 in]
      n404 = local read "light_80"() -> ()  [unwired: 1 in]
      n405 = call "DAQNavi Assistant"() -> ()  [unwired: 2 in, 18 out]
    }
    frame Enabled {
    }
  }
  n406 = while {
    stop <- w13 stop-if-true
    n407 = event shown="[13] \"btn_开始试验\": 值改变" {
      selector: _ -> [_ _ _ _ _ _ _ _ _ _ _ _ _ _ _ _ _ _ _]
      dyn-events: _ -> [_ _ _ _ _ _ _ _ _ _ _ _ _ _ _ _ _ _ _]
      timeout: _ -> [_ _ _ _ _ _ _ _ _ _ _ _ _ _ _ _ _ _ _]
      tunnel: [_ w14 w15 _ _ _ _ _ _ _ _ _ _ _ _ _ _ _ _] -> w13
      event Timeout {
        n408 = event-data() -> ()  [unwired: 1 in, 2 out]
      }
      event Panel Close {
        w14 = TRUE ("关闭？")
        n409 = event-data() -> ()  [unwired: 1 in, 3 out]
        n410 = local write "关闭？"(w14) -> ()
      }
      event "btn_关闭": Value Change {
        w15 = TRUE
        n411 = event-data() -> ()  [unwired: 1 in, 5 out]
        n412 = local write "关闭？"(w15) -> ()
      }
      event "btn_全选_1": Value Change {
        n413 = event-data() -> ("NewVal"=w17:bool)  [unwired: 1 in, 4 out]
        n414 = case shown="假" w17 {
          tunnel: [FALSE ("单选_第41路") TRUE ("单选_第41路")] -> w16
          frame False {
          }
          frame True {
          }
        }
        n415 = local write "单选_第1路"(w16) -> ()
        n416 = local write "单选_第2路"(w16) -> ()
        n417 = local write "单选_第3路"(w16) -> ()
        n418 = local write "单选_第4路"(w16) -> ()
        n419 = local write "单选_第5路"(w16) -> ()
        n420 = local write "单选_第6路"(w16) -> ()
        n421 = local write "单选_第7路"(w16) -> ()
        n422 = local write "单选_第8路"(w16) -> ()
        n423 = local write "单选_第9路"(w16) -> ()
        n424 = local write "单选_第10路"(w16) -> ()
        n425 = local write "单选_第11路"(w16) -> ()
        n426 = local write "单选_第12路"(w16) -> ()
        n427 = local write "单选_第13路"(w16) -> ()
        n428 = local write "单选_第14路"(w16) -> ()
        n429 = local write "单选_第15路"(w16) -> ()
        n430 = local write "单选_第16路"(w16) -> ()
      }
      event "btn_全选_2": Value Change {
        n431 = event-data() -> ("NewVal"=w21:bool)  [unwired: 1 in, 4 out]
        n432 = case shown="假" w21 {
          tunnel: [FALSE ("单选_第41路") TRUE ("单选_第41路")] -> w20
          frame False {
          }
          frame True {
          }
        }
        n433 = local write "单选_第17路"(w20) -> ()
        n434 = local write "单选_第18路"(w20) -> ()
        n435 = local write "单选_第19路"(w20) -> ()
        n436 = local write "单选_第20路"(w20) -> ()
        n437 = local write "单选_第21路"(w20) -> ()
        n438 = local write "单选_第22路"(w20) -> ()
        n439 = local write "单选_第23路"(w20) -> ()
        n440 = local write "单选_第24路"(w20) -> ()
        n441 = local write "单选_第25路"(w20) -> ()
        n442 = local write "单选_第26路"(w20) -> ()
        n443 = local write "单选_第27路"(w20) -> ()
        n444 = local write "单选_第28路"(w20) -> ()
        n445 = local write "单选_第29路"(w20) -> ()
        n446 = local write "单选_第30路"(w20) -> ()
        n447 = local write "单选_第31路"(w20) -> ()
        n448 = local write "单选_第32路"(w20) -> ()
      }
      event "btn_全选_3": Value Change {
        n449 = event-data() -> ("NewVal"=w25:bool)  [unwired: 1 in, 4 out]
        n450 = case shown="假" w25 {
          tunnel: [FALSE ("单选_第41路") TRUE ("单选_第41路")] -> w24
          frame False {
          }
          frame True {
          }
        }
        n451 = local write "单选_第33路"(w24) -> ()
        n452 = local write "单选_第34路"(w24) -> ()
        n453 = local write "单选_第35路"(w24) -> ()
        n454 = local write "单选_第36路"(w24) -> ()
        n455 = local write "单选_第37路"(w24) -> ()
        n456 = local write "单选_第38路"(w24) -> ()
        n457 = local write "单选_第39路"(w24) -> ()
        n458 = local write "单选_第40路"(w24) -> ()
        n459 = local write "单选_第41路"(w24) -> ()
        n460 = local write "单选_第42路"(w24) -> ()
        n461 = local write "单选_第43路"(w24) -> ()
        n462 = local write "单选_第44路"(w24) -> ()
        n463 = local write "单选_第45路"(w24) -> ()
        n464 = local write "单选_第46路"(w24) -> ()
        n465 = local write "单选_第47路"(w24) -> ()
        n466 = local write "单选_第48路"(w24) -> ()
      }
      event "btn_全选_4": Value Change {
        n467 = event-data() -> ("NewVal"=w29:bool)  [unwired: 1 in, 4 out]
        n468 = case shown="假" w29 {
          tunnel: [FALSE ("单选_第41路") TRUE ("单选_第41路")] -> w28
          frame False {
          }
          frame True {
          }
        }
        n469 = local write "单选_第49路"(w28) -> ()
        n470 = local write "单选_第50路"(w28) -> ()
        n471 = local write "单选_第51路"(w28) -> ()
        n472 = local write "单选_第52路"(w28) -> ()
        n473 = local write "单选_第53路"(w28) -> ()
        n474 = local write "单选_第54路"(w28) -> ()
        n475 = local write "单选_第55路"(w28) -> ()
        n476 = local write "单选_第56路"(w28) -> ()
        n477 = local write "单选_第57路"(w28) -> ()
        n478 = local write "单选_第58路"(w28) -> ()
        n479 = local write "单选_第59路"(w28) -> ()
        n480 = local write "单选_第60路"(w28) -> ()
        n481 = local write "单选_第61路"(w28) -> ()
        n482 = local write "单选_第62路"(w28) -> ()
        n483 = local write "单选_第63路"(w28) -> ()
        n484 = local write "单选_第64路"(w28) -> ()
      }
      event "btn_全选_5": Value Change {
        n485 = event-data() -> ("NewVal"=w33:bool)  [unwired: 1 in, 4 out]
        n486 = case shown="假" w33 {
          tunnel: [FALSE ("单选_第41路") TRUE ("单选_第41路")] -> w32
          frame False {
          }
          frame True {
          }
        }
        n487 = local write "单选_第71路"(w32) -> ()
        n488 = local write "单选_第79路"(w32) -> ()
        n489 = local write "单选_第65路"(w32) -> ()
        n490 = local write "单选_第66路"(w32) -> ()
        n491 = local write "单选_第67路"(w32) -> ()
        n492 = local write "单选_第68路"(w32) -> ()
        n493 = local write "单选_第69路"(w32) -> ()
        n494 = local write "单选_第70路"(w32) -> ()
        n495 = local write "单选_第72路"(w32) -> ()
        n496 = local write "单选_第73路"(w32) -> ()
        n497 = local write "单选_第74路"(w32) -> ()
        n498 = local write "单选_第75路"(w32) -> ()
        n499 = local write "单选_第76路"(w32) -> ()
        n500 = local write "单选_第77路"(w32) -> ()
        n501 = local write "单选_第78路"(w32) -> ()
        n502 = local write "单选_第80路"(w32) -> ()
      }
      event "btn_置1_1": Value Change {
        n503 = event-data() -> ("NewVal"=w37:bool)  [unwired: 1 in, 4 out]
        n504 = case shown="假" w37 {
          tunnel: [enum16{"0", "1"}."0" ("输入值_41") enum16{"0", "1"}."1" ("输入值_41")] -> w36
          frame False {
          }
          frame True {
          }
        }
        n505 = local write "输入值_1"(w36) -> ()
        n506 = local write "输入值_2"(w36) -> ()
        n507 = local write "输入值_3"(w36) -> ()
        n508 = local write "输入值_4"(w36) -> ()
        n509 = local write "输入值_5"(w36) -> ()
        n510 = local write "输入值_6"(w36) -> ()
        n511 = local write "输入值_7"(w36) -> ()
        n512 = local write "输入值_8"(w36) -> ()
        n513 = local write "输入值_9"(w36) -> ()
        n514 = local write "输入值_10"(w36) -> ()
        n515 = local write "输入值_11"(w36) -> ()
        n516 = local write "输入值_12"(w36) -> ()
        n517 = local write "输入值_13"(w36) -> ()
        n518 = local write "输入值_14"(w36) -> ()
        n519 = local write "输入值_15"(w36) -> ()
        n520 = local write "输入值_16"(w36) -> ()
      }
      event "btn_置1_2": Value Change {
        n521 = event-data() -> ("NewVal"=w41:bool)  [unwired: 1 in, 4 out]
        n522 = case shown="假" w41 {
          tunnel: [enum16{"0", "1"}."0" ("输入值_41") enum16{"0", "1"}."1" ("输入值_41")] -> w40
          frame False {
          }
          frame True {
          }
        }
        n523 = local write "输入值_17"(w40) -> ()
        n524 = local write "输入值_18"(w40) -> ()
        n525 = local write "输入值_19"(w40) -> ()
        n526 = local write "输入值_20"(w40) -> ()
        n527 = local write "输入值_21"(w40) -> ()
        n528 = local write "输入值_22"(w40) -> ()
        n529 = local write "输入值_23"(w40) -> ()
        n530 = local write "输入值_24"(w40) -> ()
        n531 = local write "输入值_25"(w40) -> ()
        n532 = local write "输入值_26"(w40) -> ()
        n533 = local write "输入值_27"(w40) -> ()
        n534 = local write "输入值_28"(w40) -> ()
        n535 = local write "输入值_29"(w40) -> ()
        n536 = local write "输入值_30"(w40) -> ()
        n537 = local write "输入值_31"(w40) -> ()
        n538 = local write "输入值_32"(w40) -> ()
      }
      event "btn_置1_3": Value Change {
        n539 = event-data() -> ("NewVal"=w45:bool)  [unwired: 1 in, 4 out]
        n540 = case shown="假" w45 {
          tunnel: [enum16{"0", "1"}."0" ("输入值_41") enum16{"0", "1"}."1" ("输入值_41")] -> w44
          frame False {
          }
          frame True {
          }
        }
        n541 = local write "输入值_33"(w44) -> ()
        n542 = local write "输入值_34"(w44) -> ()
        n543 = local write "输入值_35"(w44) -> ()
        n544 = local write "输入值_36"(w44) -> ()
        n545 = local write "输入值_37"(w44) -> ()
        n546 = local write "输入值_38"(w44) -> ()
        n547 = local write "输入值_39"(w44) -> ()
        n548 = local write "输入值_40"(w44) -> ()
        n549 = local write "输入值_41"(w44) -> ()
        n550 = local write "输入值_42"(w44) -> ()
        n551 = local write "输入值_43"(w44) -> ()
        n552 = local write "输入值_44"(w44) -> ()
        n553 = local write "输入值_45"(w44) -> ()
        n554 = local write "输入值_46"(w44) -> ()
        n555 = local write "输入值_47"(w44) -> ()
        n556 = local write "输入值_48"(w44) -> ()
      }
      event "btn_置1_4": Value Change {
        n557 = event-data() -> ("NewVal"=w49:bool)  [unwired: 1 in, 4 out]
        n558 = case shown="假" w49 {
          tunnel: [enum16{"0", "1"}."0" ("输入值_41") enum16{"0", "1"}."1" ("输入值_41")] -> w48
          frame False {
          }
          frame True {
          }
        }
        n559 = local write "输入值_49"(w48) -> ()
        n560 = local write "输入值_50"(w48) -> ()
        n561 = local write "输入值_51"(w48) -> ()
        n562 = local write "输入值_52"(w48) -> ()
        n563 = local write "输入值_53"(w48) -> ()
        n564 = local write "输入值_54"(w48) -> ()
        n565 = local write "输入值_55"(w48) -> ()
        n566 = local write "输入值_56"(w48) -> ()
        n567 = local write "输入值_57"(w48) -> ()
        n568 = local write "输入值_58"(w48) -> ()
        n569 = local write "输入值_59"(w48) -> ()
        n570 = local write "输入值_60"(w48) -> ()
        n571 = local write "输入值_61"(w48) -> ()
        n572 = local write "输入值_62"(w48) -> ()
        n573 = local write "输入值_63"(w48) -> ()
        n574 = local write "输入值_64"(w48) -> ()
      }
      event "btn_置1_5": Value Change {
        n575 = event-data() -> ("NewVal"=w53:bool)  [unwired: 1 in, 4 out]
        n576 = case shown="假" w53 {
          tunnel: [enum16{"0", "1"}."0" ("输入值_41") enum16{"0", "1"}."1" ("输入值_41")] -> w52
          frame False {
          }
          frame True {
          }
        }
        n577 = local write "输入值_65"(w52) -> ()
        n578 = local write "输入值_66"(w52) -> ()
        n579 = local write "输入值_67"(w52) -> ()
        n580 = local write "输入值_68"(w52) -> ()
        n581 = local write "输入值_69"(w52) -> ()
        n582 = local write "输入值_70"(w52) -> ()
        n583 = local write "输入值_71"(w52) -> ()
        n584 = local write "输入值_72"(w52) -> ()
        n585 = local write "输入值_73"(w52) -> ()
        n586 = local write "输入值_74"(w52) -> ()
        n587 = local write "输入值_75"(w52) -> ()
        n588 = local write "输入值_76"(w52) -> ()
        n589 = local write "输入值_77"(w52) -> ()
        n590 = local write "输入值_78"(w52) -> ()
        n591 = local write "输入值_79"(w52) -> ()
        n592 = local write "输入值_80"(w52) -> ()
      }
      event "btn_开始试验": Value Change {
        n593 = event-data() -> ()  [unwired: 1 in, 5 out]
        n594 = stacked-sequence {
          frame #0 {
            w57 = 0 ("同步_A1")
            n595 = stacked-sequence {
              tunnel: [w83 _ _ _ _] -> w79
              tunnel: [w82 _ _ _ _] -> w63
              tunnel: [_ w117 _ _ _] -> w77
              tunnel: [_ w116 _ _ _] -> w62
              tunnel: [_ _ w151 _ _] -> w75
              tunnel: [_ _ w150 _ _] -> w61
              tunnel: [_ _ _ w185 _] -> w73
              tunnel: [_ _ _ w184 _] -> w60
              tunnel: [_ _ _ _ w219] -> w71
              tunnel: [_ _ _ _ w218] -> w59
              frame #0 {
                n596 = local read "单选_第1路"() -> (w100:bool)
                n597 = local read "单选_第2路"() -> (w101:bool)
                n598 = local read "单选_第3路"() -> (w102:bool)
                n599 = local read "单选_第4路"() -> (w103:bool)
                n600 = local read "单选_第5路"() -> (w104:bool)
                n601 = local read "单选_第6路"() -> (w105:bool)
                n602 = local read "单选_第7路"() -> (w106:bool)
                n603 = local read "单选_第8路"() -> (w107:bool)
                n604 = local read "单选_第9路"() -> (w108:bool)
                n605 = local read "单选_第10路"() -> (w109:bool)
                n606 = local read "单选_第11路"() -> (w110:bool)
                n607 = local read "单选_第12路"() -> (w111:bool)
                n608 = local read "单选_第13路"() -> (w112:bool)
                n609 = local read "单选_第14路"() -> (w113:bool)
                n610 = local read "单选_第15路"() -> (w114:bool)
                n611 = local read "单选_第16路"() -> (w115:bool)
                n612 = local read "输入值_1"() -> (w84:enum16{"0", "1"})
                n613 = local read "输入值_2"() -> (w85:enum16{"0", "1"})
                n614 = local read "输入值_3"() -> (w86:enum16{"0", "1"})
                n615 = local read "输入值_4"() -> (w87:enum16{"0", "1"})
                n616 = local read "输入值_5"() -> (w88:enum16{"0", "1"})
                n617 = local read "输入值_6"() -> (w89:enum16{"0", "1"})
                n618 = local read "输入值_7"() -> (w90:enum16{"0", "1"})
                n619 = local read "输入值_8"() -> (w91:enum16{"0", "1"})
                n620 = local read "输入值_9"() -> (w92:enum16{"0", "1"})
                n621 = local read "输入值_10"() -> (w93:enum16{"0", "1"})
                n622 = local read "输入值_11"() -> (w94:enum16{"0", "1"})
                n623 = local read "输入值_12"() -> (w95:enum16{"0", "1"})
                n624 = local read "输入值_13"() -> (w96:enum16{"0", "1"})
                n625 = local read "输入值_14"() -> (w97:enum16{"0", "1"})
                n626 = local read "输入值_15"() -> (w98:enum16{"0", "1"})
                n627 = local read "输入值_16"() -> (w99:enum16{"0", "1"})
                n628 = Build Array(w100, w101, w102, w103, w104, w105, w106, w107, w108, w109, w110, w111, w112, w113, w114, w115) -> (w83:bool[])
                n629 = Build Array(w84, w85, w86, w87, w88, w89, w90, w91, w92, w93, w94, w95, w96, w97, w98, w99) -> (w82:enum16{"0", "1"}[])
              }
              frame #1 {
                n630 = local read "单选_第17路"() -> (w134:bool)
                n631 = local read "单选_第18路"() -> (w135:bool)
                n632 = local read "单选_第19路"() -> (w136:bool)
                n633 = local read "单选_第20路"() -> (w137:bool)
                n634 = local read "单选_第21路"() -> (w138:bool)
                n635 = local read "单选_第22路"() -> (w139:bool)
                n636 = local read "单选_第23路"() -> (w140:bool)
                n637 = local read "单选_第24路"() -> (w141:bool)
                n638 = local read "单选_第25路"() -> (w142:bool)
                n639 = local read "单选_第26路"() -> (w143:bool)
                n640 = local read "单选_第27路"() -> (w144:bool)
                n641 = local read "单选_第28路"() -> (w145:bool)
                n642 = local read "单选_第29路"() -> (w146:bool)
                n643 = local read "单选_第30路"() -> (w147:bool)
                n644 = local read "单选_第31路"() -> (w148:bool)
                n645 = local read "单选_第32路"() -> (w149:bool)
                n646 = local read "输入值_17"() -> (w118:enum16{"0", "1"})
                n647 = local read "输入值_18"() -> (w119:enum16{"0", "1"})
                n648 = local read "输入值_19"() -> (w120:enum16{"0", "1"})
                n649 = local read "输入值_20"() -> (w121:enum16{"0", "1"})
                n650 = local read "输入值_21"() -> (w122:enum16{"0", "1"})
                n651 = local read "输入值_22"() -> (w123:enum16{"0", "1"})
                n652 = local read "输入值_23"() -> (w124:enum16{"0", "1"})
                n653 = local read "输入值_24"() -> (w125:enum16{"0", "1"})
                n654 = local read "输入值_25"() -> (w126:enum16{"0", "1"})
                n655 = local read "输入值_26"() -> (w127:enum16{"0", "1"})
                n656 = local read "输入值_27"() -> (w128:enum16{"0", "1"})
                n657 = local read "输入值_28"() -> (w129:enum16{"0", "1"})
                n658 = local read "输入值_29"() -> (w130:enum16{"0", "1"})
                n659 = local read "输入值_30"() -> (w131:enum16{"0", "1"})
                n660 = local read "输入值_31"() -> (w132:enum16{"0", "1"})
                n661 = local read "输入值_32"() -> (w133:enum16{"0", "1"})
                n662 = Build Array(w134, w135, w136, w137, w138, w139, w140, w141, w142, w143, w144, w145, w146, w147, w148, w149) -> (w117:bool[])
                n663 = Build Array(w118, w119, w120, w121, w122, w123, w124, w125, w126, w127, w128, w129, w130, w131, w132, w133) -> (w116:enum16{"0", "1"}[])
              }
              frame #2 {
                n664 = local read "单选_第33路"() -> (w168:bool)
                n665 = local read "单选_第34路"() -> (w169:bool)
                n666 = local read "单选_第35路"() -> (w170:bool)
                n667 = local read "单选_第36路"() -> (w171:bool)
                n668 = local read "单选_第37路"() -> (w172:bool)
                n669 = local read "单选_第38路"() -> (w173:bool)
                n670 = local read "单选_第39路"() -> (w174:bool)
                n671 = local read "单选_第40路"() -> (w175:bool)
                n672 = local read "单选_第41路"() -> (w176:bool)
                n673 = local read "单选_第42路"() -> (w177:bool)
                n674 = local read "单选_第43路"() -> (w178:bool)
                n675 = local read "单选_第44路"() -> (w179:bool)
                n676 = local read "单选_第45路"() -> (w180:bool)
                n677 = local read "单选_第46路"() -> (w181:bool)
                n678 = local read "单选_第47路"() -> (w182:bool)
                n679 = local read "单选_第48路"() -> (w183:bool)
                n680 = local read "输入值_33"() -> (w152:enum16{"0", "1"})
                n681 = local read "输入值_34"() -> (w153:enum16{"0", "1"})
                n682 = local read "输入值_35"() -> (w154:enum16{"0", "1"})
                n683 = local read "输入值_36"() -> (w155:enum16{"0", "1"})
                n684 = local read "输入值_37"() -> (w156:enum16{"0", "1"})
                n685 = local read "输入值_38"() -> (w157:enum16{"0", "1"})
                n686 = local read "输入值_39"() -> (w158:enum16{"0", "1"})
                n687 = local read "输入值_40"() -> (w159:enum16{"0", "1"})
                n688 = local read "输入值_41"() -> (w160:enum16{"0", "1"})
                n689 = local read "输入值_42"() -> (w161:enum16{"0", "1"})
                n690 = local read "输入值_43"() -> (w162:enum16{"0", "1"})
                n691 = local read "输入值_44"() -> (w163:enum16{"0", "1"})
                n692 = local read "输入值_45"() -> (w164:enum16{"0", "1"})
                n693 = local read "输入值_46"() -> (w165:enum16{"0", "1"})
                n694 = local read "输入值_47"() -> (w166:enum16{"0", "1"})
                n695 = local read "输入值_48"() -> (w167:enum16{"0", "1"})
                n696 = Build Array(w152, w153, w154, w155, w156, w157, w158, w159, w160, w161, w162, w163, w164, w165, w166, w167) -> (w150:enum16{"0", "1"}[])
                n697 = Build Array(w168, w169, w170, w171, w172, w173, w174, w175, w176, w177, w178, w179, w180, w181, w182, w183) -> (w151:bool[])
              }
              frame #3 {
                n698 = local read "单选_第49路"() -> (w202:bool)
                n699 = local read "单选_第50路"() -> (w203:bool)
                n700 = local read "单选_第51路"() -> (w204:bool)
                n701 = local read "单选_第52路"() -> (w205:bool)
                n702 = local read "单选_第53路"() -> (w206:bool)
                n703 = local read "单选_第54路"() -> (w207:bool)
                n704 = local read "单选_第55路"() -> (w208:bool)
                n705 = local read "单选_第56路"() -> (w209:bool)
                n706 = local read "单选_第57路"() -> (w210:bool)
                n707 = local read "单选_第58路"() -> (w211:bool)
                n708 = local read "单选_第59路"() -> (w212:bool)
                n709 = local read "单选_第60路"() -> (w213:bool)
                n710 = local read "单选_第61路"() -> (w214:bool)
                n711 = local read "单选_第62路"() -> (w215:bool)
                n712 = local read "单选_第63路"() -> (w216:bool)
                n713 = local read "单选_第64路"() -> (w217:bool)
                n714 = local read "输入值_49"() -> (w186:enum16{"0", "1"})
                n715 = local read "输入值_50"() -> (w187:enum16{"0", "1"})
                n716 = local read "输入值_51"() -> (w188:enum16{"0", "1"})
                n717 = local read "输入值_52"() -> (w189:enum16{"0", "1"})
                n718 = local read "输入值_53"() -> (w190:enum16{"0", "1"})
                n719 = local read "输入值_54"() -> (w191:enum16{"0", "1"})
                n720 = local read "输入值_55"() -> (w192:enum16{"0", "1"})
                n721 = local read "输入值_56"() -> (w193:enum16{"0", "1"})
                n722 = local read "输入值_57"() -> (w194:enum16{"0", "1"})
                n723 = local read "输入值_58"() -> (w195:enum16{"0", "1"})
                n724 = local read "输入值_59"() -> (w196:enum16{"0", "1"})
                n725 = local read "输入值_60"() -> (w197:enum16{"0", "1"})
                n726 = local read "输入值_61"() -> (w198:enum16{"0", "1"})
                n727 = local read "输入值_62"() -> (w199:enum16{"0", "1"})
                n728 = local read "输入值_63"() -> (w200:enum16{"0", "1"})
                n729 = local read "输入值_64"() -> (w201:enum16{"0", "1"})
                n730 = Build Array(w202, w203, w204, w205, w206, w207, w208, w209, w210, w211, w212, w213, w214, w215, w216, w217) -> (w185:bool[])
                n731 = Build Array(w186, w187, w188, w189, w190, w191, w192, w193, w194, w195, w196, w197, w198, w199, w200, w201) -> (w184:enum16{"0", "1"}[])
              }
              frame #4 {
                n732 = local read "单选_第71路"() -> (w242:bool)
                n733 = local read "单选_第79路"() -> (w250:bool)
                n734 = local read "单选_第65路"() -> (w236:bool)
                n735 = local read "单选_第66路"() -> (w237:bool)
                n736 = local read "单选_第67路"() -> (w238:bool)
                n737 = local read "单选_第68路"() -> (w239:bool)
                n738 = local read "单选_第69路"() -> (w240:bool)
                n739 = local read "单选_第70路"() -> (w241:bool)
                n740 = local read "单选_第72路"() -> (w243:bool)
                n741 = local read "单选_第73路"() -> (w244:bool)
                n742 = local read "单选_第74路"() -> (w245:bool)
                n743 = local read "单选_第75路"() -> (w246:bool)
                n744 = local read "单选_第76路"() -> (w247:bool)
                n745 = local read "单选_第77路"() -> (w248:bool)
                n746 = local read "单选_第78路"() -> (w249:bool)
                n747 = local read "单选_第80路"() -> (w251:bool)
                n748 = local read "输入值_65"() -> (w220:enum16{"0", "1"})
                n749 = local read "输入值_66"() -> (w221:enum16{"0", "1"})
                n750 = local read "输入值_67"() -> (w222:enum16{"0", "1"})
                n751 = local read "输入值_68"() -> (w223:enum16{"0", "1"})
                n752 = local read "输入值_69"() -> (w224:enum16{"0", "1"})
                n753 = local read "输入值_70"() -> (w225:enum16{"0", "1"})
                n754 = local read "输入值_71"() -> (w226:enum16{"0", "1"})
                n755 = local read "输入值_72"() -> (w227:enum16{"0", "1"})
                n756 = local read "输入值_73"() -> (w228:enum16{"0", "1"})
                n757 = local read "输入值_74"() -> (w229:enum16{"0", "1"})
                n758 = local read "输入值_75"() -> (w230:enum16{"0", "1"})
                n759 = local read "输入值_76"() -> (w231:enum16{"0", "1"})
                n760 = local read "输入值_77"() -> (w232:enum16{"0", "1"})
                n761 = local read "输入值_78"() -> (w233:enum16{"0", "1"})
                n762 = local read "输入值_79"() -> (w234:enum16{"0", "1"})
                n763 = local read "输入值_80"() -> (w235:enum16{"0", "1"})
                n764 = Build Array(w220, w221, w222, w223, w224, w225, w226, w227, w228, w229, w230, w231, w232, w233, w234, w235) -> (w218:enum16{"0", "1"}[])
                n765 = Build Array(w236, w237, w238, w239, w240, w241, w242, w243, w244, w245, w246, w247, w248, w249, w250, w251) -> (w219:bool[])
              }
            }
            n766 = local read "数组_选择?"() -> (w81:bool[][])
            n767 = local read "数组_输入值"() -> (w64:enum16{"0", "1"}[][])
            n768 = Replace Array Subset(array=w81, new element #1=w79, index (row) #1=0 ("索引 (行)"), new element #2=w77, index (row) #2=1 ("索引 (行)"), new element #3=w75, index (row) #3=2 ("索引 (行)"), new element #4=w73, index (row) #4=3 ("索引 (行)"), new element #5=w71, index (row) #5=4 ("索引 (行)")) -> (w70:bool[][])  [unwired: 5 in]
            n769 = local write "测试结论"("") -> ()
            n770 = local write "同步_A1"(w57) -> ()
            n771 = local write "同步_A2"(w57) -> ()
            n772 = Replace Array Subset(array=w64, new element #1=w63, index (row) #1=0 ("索引 (行)"), new element #2=w62, index (row) #2=1 ("索引 (行)"), new element #3=w61, index (row) #3=2 ("索引 (行)"), new element #4=w60, index (row) #4=3 ("索引 (行)"), new element #5=w59, index (row) #5=4 ("索引 (行)")) -> (w58:enum16{"0", "1"}[][])  [unwired: 5 in]
            n773 = local write "数组_输入值"(w58) -> ()
            n774 = local write "数组_选择?"(w70) -> ()
          }
          frame #1 {
            w252 = cluster{u32, u32}[] [{9868950, 9868950}]
            n775 = property on="light_1" class="Bool (严格)"("Colors [4]"=w252) -> ()  [unwired: 2 in, 2 out]
            n776 = property on="light_2" class="Bool (严格)"("Colors [4]"=w252) -> ()  [unwired: 2 in, 2 out]
            n777 = property on="light_3" class="Bool (严格)"("Colors [4]"=w252) -> ()  [unwired: 2 in, 2 out]
            n778 = property on="light_4" class="Bool (严格)"("Colors [4]"=w252) -> ()  [unwired: 2 in, 2 out]
            n779 = property on="light_5" class="Bool (严格)"("Colors [4]"=w252) -> ()  [unwired: 2 in, 2 out]
            n780 = property on="light_6" class="Bool (严格)"("Colors [4]"=w252) -> ()  [unwired: 2 in, 2 out]
            n781 = property on="light_7" class="Bool (严格)"("Colors [4]"=w252) -> ()  [unwired: 2 in, 2 out]
            n782 = property on="light_8" class="Bool (严格)"("Colors [4]"=w252) -> ()  [unwired: 2 in, 2 out]
            n783 = property on="light_9" class="Bool (严格)"("Colors [4]"=w252) -> ()  [unwired: 2 in, 2 out]
            n784 = property on="light_10" class="Bool (严格)"("Colors [4]"=w252) -> ()  [unwired: 2 in, 2 out]
            n785 = property on="light_11" class="Bool (严格)"("Colors [4]"=w252) -> ()  [unwired: 2 in, 2 out]
            n786 = property on="light_12" class="Bool (严格)"("Colors [4]"=w252) -> ()  [unwired: 2 in, 2 out]
            n787 = property on="light_13" class="Bool (严格)"("Colors [4]"=w252) -> ()  [unwired: 2 in, 2 out]
            n788 = property on="light_14" class="Bool (严格)"("Colors [4]"=w252) -> ()  [unwired: 2 in, 2 out]
            n789 = property on="light_15" class="Bool (严格)"("Colors [4]"=w252) -> ()  [unwired: 2 in, 2 out]
            n790 = property on="light_16" class="Bool (严格)"("Colors [4]"=w252) -> ()  [unwired: 2 in, 2 out]
            n791 = property on="light_17" class="Bool (严格)"("Colors [4]"=w252) -> ()  [unwired: 2 in, 2 out]
            n792 = property on="light_18" class="Bool (严格)"("Colors [4]"=w252) -> ()  [unwired: 2 in, 2 out]
            n793 = property on="light_19" class="Bool (严格)"("Colors [4]"=w252) -> ()  [unwired: 2 in, 2 out]
            n794 = property on="light_20" class="Bool (严格)"("Colors [4]"=w252) -> ()  [unwired: 2 in, 2 out]
            n795 = property on="light_21" class="Bool (严格)"("Colors [4]"=w252) -> ()  [unwired: 2 in, 2 out]
            n796 = property on="light_22" class="Bool (严格)"("Colors [4]"=w252) -> ()  [unwired: 2 in, 2 out]
            n797 = property on="light_23" class="Bool (严格)"("Colors [4]"=w252) -> ()  [unwired: 2 in, 2 out]
            n798 = property on="light_24" class="Bool (严格)"("Colors [4]"=w252) -> ()  [unwired: 2 in, 2 out]
            n799 = property on="light_25" class="Bool (严格)"("Colors [4]"=w252) -> ()  [unwired: 2 in, 2 out]
            n800 = property on="light_26" class="Bool (严格)"("Colors [4]"=w252) -> ()  [unwired: 2 in, 2 out]
            n801 = property on="light_27" class="Bool (严格)"("Colors [4]"=w252) -> ()  [unwired: 2 in, 2 out]
            n802 = property on="light_28" class="Bool (严格)"("Colors [4]"=w252) -> ()  [unwired: 2 in, 2 out]
            n803 = property on="light_29" class="Bool (严格)"("Colors [4]"=w252) -> ()  [unwired: 2 in, 2 out]
            n804 = property on="light_30" class="Bool (严格)"("Colors [4]"=w252) -> ()  [unwired: 2 in, 2 out]
            n805 = property on="light_31" class="Bool (严格)"("Colors [4]"=w252) -> ()  [unwired: 2 in, 2 out]
            n806 = property on="light_32" class="Bool (严格)"("Colors [4]"=w252) -> ()  [unwired: 2 in, 2 out]
            n807 = property on="light_33" class="Bool (严格)"("Colors [4]"=w252) -> ()  [unwired: 2 in, 2 out]
            n808 = property on="light_34" class="Bool (严格)"("Colors [4]"=w252) -> ()  [unwired: 2 in, 2 out]
            n809 = property on="light_35" class="Bool (严格)"("Colors [4]"=w252) -> ()  [unwired: 2 in, 2 out]
            n810 = property on="light_36" class="Bool (严格)"("Colors [4]"=w252) -> ()  [unwired: 2 in, 2 out]
            n811 = property on="light_37" class="Bool (严格)"("Colors [4]"=w252) -> ()  [unwired: 2 in, 2 out]
            n812 = property on="light_38" class="Bool (严格)"("Colors [4]"=w252) -> ()  [unwired: 2 in, 2 out]
            n813 = property on="light_39" class="Bool (严格)"("Colors [4]"=w252) -> ()  [unwired: 2 in, 2 out]
            n814 = property on="light_40" class="Bool (严格)"("Colors [4]"=w252) -> ()  [unwired: 2 in, 2 out]
            n815 = property on="light_41" class="Bool (严格)"("Colors [4]"=w252) -> ()  [unwired: 2 in, 2 out]
            n816 = property on="light_42" class="Bool (严格)"("Colors [4]"=w252) -> ()  [unwired: 2 in, 2 out]
            n817 = property on="light_43" class="Bool (严格)"("Colors [4]"=w252) -> ()  [unwired: 2 in, 2 out]
            n818 = property on="light_44" class="Bool (严格)"("Colors [4]"=w252) -> ()  [unwired: 2 in, 2 out]
            n819 = property on="light_45" class="Bool (严格)"("Colors [4]"=w252) -> ()  [unwired: 2 in, 2 out]
            n820 = property on="light_46" class="Bool (严格)"("Colors [4]"=w252) -> ()  [unwired: 2 in, 2 out]
            n821 = property on="light_47" class="Bool (严格)"("Colors [4]"=w252) -> ()  [unwired: 2 in, 2 out]
            n822 = property on="light_48" class="Bool (严格)"("Colors [4]"=w252) -> ()  [unwired: 2 in, 2 out]
            n823 = property on="light_49" class="Bool (严格)"("Colors [4]"=w252) -> ()  [unwired: 2 in, 2 out]
            n824 = property on="light_50" class="Bool (严格)"("Colors [4]"=w252) -> ()  [unwired: 2 in, 2 out]
            n825 = property on="light_51" class="Bool (严格)"("Colors [4]"=w252) -> ()  [unwired: 2 in, 2 out]
            n826 = property on="light_52" class="Bool (严格)"("Colors [4]"=w252) -> ()  [unwired: 2 in, 2 out]
            n827 = property on="light_53" class="Bool (严格)"("Colors [4]"=w252) -> ()  [unwired: 2 in, 2 out]
            n828 = property on="light_54" class="Bool (严格)"("Colors [4]"=w252) -> ()  [unwired: 2 in, 2 out]
            n829 = property on="light_55" class="Bool (严格)"("Colors [4]"=w252) -> ()  [unwired: 2 in, 2 out]
            n830 = property on="light_56" class="Bool (严格)"("Colors [4]"=w252) -> ()  [unwired: 2 in, 2 out]
            n831 = property on="light_57" class="Bool (严格)"("Colors [4]"=w252) -> ()  [unwired: 2 in, 2 out]
            n832 = property on="light_58" class="Bool (严格)"("Colors [4]"=w252) -> ()  [unwired: 2 in, 2 out]
            n833 = property on="light_59" class="Bool (严格)"("Colors [4]"=w252) -> ()  [unwired: 2 in, 2 out]
            n834 = property on="light_60" class="Bool (严格)"("Colors [4]"=w252) -> ()  [unwired: 2 in, 2 out]
            n835 = property on="light_61" class="Bool (严格)"("Colors [4]"=w252) -> ()  [unwired: 2 in, 2 out]
            n836 = property on="light_62" class="Bool (严格)"("Colors [4]"=w252) -> ()  [unwired: 2 in, 2 out]
            n837 = property on="light_63" class="Bool (严格)"("Colors [4]"=w252) -> ()  [unwired: 2 in, 2 out]
            n838 = property on="light_64" class="Bool (严格)"("Colors [4]"=w252) -> ()  [unwired: 2 in, 2 out]
            n839 = property on="light_65" class="Bool (严格)"("Colors [4]"=w252) -> ()  [unwired: 2 in, 2 out]
            n840 = property on="light_66" class="Bool (严格)"("Colors [4]"=w252) -> ()  [unwired: 2 in, 2 out]
            n841 = property on="light_67" class="Bool (严格)"("Colors [4]"=w252) -> ()  [unwired: 2 in, 2 out]
            n842 = property on="light_68" class="Bool (严格)"("Colors [4]"=w252) -> ()  [unwired: 2 in, 2 out]
            n843 = property on="light_69" class="Bool (严格)"("Colors [4]"=w252) -> ()  [unwired: 2 in, 2 out]
            n844 = property on="light_70" class="Bool (严格)"("Colors [4]"=w252) -> ()  [unwired: 2 in, 2 out]
            n845 = property on="light_71" class="Bool (严格)"("Colors [4]"=w252) -> ()  [unwired: 2 in, 2 out]
            n846 = property on="light_72" class="Bool (严格)"("Colors [4]"=w252) -> ()  [unwired: 2 in, 2 out]
            n847 = property on="light_73" class="Bool (严格)"("Colors [4]"=w252) -> ()  [unwired: 2 in, 2 out]
            n848 = property on="light_74" class="Bool (严格)"("Colors [4]"=w252) -> ()  [unwired: 2 in, 2 out]
            n849 = property on="light_75" class="Bool (严格)"("Colors [4]"=w252) -> ()  [unwired: 2 in, 2 out]
            n850 = property on="light_76" class="Bool (严格)"("Colors [4]"=w252) -> ()  [unwired: 2 in, 2 out]
            n851 = property on="light_77" class="Bool (严格)"("Colors [4]"=w252) -> ()  [unwired: 2 in, 2 out]
            n852 = property on="light_78" class="Bool (严格)"("Colors [4]"=w252) -> ()  [unwired: 2 in, 2 out]
            n853 = property on="light_79" class="Bool (严格)"("Colors [4]"=w252) -> ()  [unwired: 2 in, 2 out]
            n854 = property on="light_80" class="Bool (严格)"("Colors [4]"=w252) -> ()  [unwired: 2 in, 2 out]
            n855 = Initialize Array("", 16 ("维数大小"), 4 ("维数大小")) -> (w256:string[][])
            n856 = local write "D_IN_1"(w256) -> ()
            n857 = local write "D_IN_2"(w256) -> ()
            n858 = local write "D_IN_3"(w256) -> ()
            n859 = local write "D_IN_4"(w256) -> ()
            n860 = local write "D_IN_5"(w256) -> ()
          }
          frame #2 {
            n861 = local read "保持输出"() -> (w257:bool)
            n862 = case shown="假" w257 {
              frame False {
                n863 = property on="保持输出" class="Bool (严格)"("DisabledEnum"=T1."Disabled and Grayed Out" ("禁用")) -> ()  [unwired: 2 in, 2 out]
              }
              frame True {
                n864 = local read "数组_选择?"() -> (w259:bool[][])
                n865 = for {
                  tunnel: w259 -> [w263] mode=indexing
                  i -> [w261]
                  stop <- w260 stop-if-true
                  n866 = Or Array Elements(Boolean array=w263) -> (logical OR=w262:bool)
                  n867 = case shown="真" w262 {
                    tunnel: w261 -> [_ w265]
                    tunnel: [FALSE TRUE] -> w260
                    frame False {
                    }
                    frame True {
                      n868 = local write "同步_A1"(w265) -> ()
                      n869 = Increment(x=w265) -> (x+1=w269:i32)
                      n870 = Format Into String(format string="保持第%d组数据输出" ("格式字符串"), w269) -> (resulting string=w268:string)  [unwired: 2 in, 1 out]
                      n871 = call "显示对话框信息5"("Message"=w268) -> ("是"=w266:bool)  [unwired: 9 in, 1 out]
                      n872 = case shown="真" w266 {
                        tunnel: w265 -> [_ w271]
                        frame False {
                        }
                        frame True {
                          n873 = stacked-sequence {
                            tunnel: w271 -> [w272 _]
                            frame #0 {
                              n874 = for {
                                N: 5 -> [_]
                                tunnel: w272 -> [w275]
                                i -> [w274]
                                n875 = Not Equal?(x=w275, y=w274) -> (x != y?=w276:bool)
                                n876 = case shown="真" w276 {
                                tunnel: w274 -> [_ w280]
                                frame False {
                                }
                                frame True {
                                n877 = local read "数组_选择?"() -> (w282:bool[][])
                                n878 = Initialize Array(FALSE, 16 ("维数大小")) -> (w277:bool[])
                                n879 = Replace Array Subset(array=w282, new element=w277, index (row)=w280) -> (w281:bool[][])  [unwired: 1 in]
                                n880 = local write "数组_选择?"(w281) -> ()
                                }
                                }
                              }
                            }
                            frame #1 {
                              n881 = property on="btn_开始试验" class="Bool"("DisabledEnum"=T1."Disabled and Grayed Out" ("禁用")) -> ()  [unwired: 2 in, 2 out]
                            }
                          }
                        }
                      }
                      n882 = local write "保持输出"(w266) -> ()
                    }
                  }
                }
              }
            }
          }
          frame #3 {
            n883 = local read "数组_选择?"() -> (w285:bool[][])
            n884 = Or Array Elements(Boolean array=w285) -> (logical OR=w284:bool)
            n885 = case shown="真" w284 {
              frame False {
                n886 = call "显示对话框信息"("Message"="请选择数字量输入路数") -> ()  [unwired: 9 in, 2 out]
              }
              frame True {
                w288 = "DIStart" ("名称（未命名）")
                n887 = Obtain Notifier(name (unnamed)=w288, notification data type=w288) -> (notifier out=w287:refnum<notifier>)  [unwired: 2 in, 2 out]
                n888 = Send Notification(notification="DInput" ("通知"), notifier=w287) -> ()  [unwired: 1 in, 2 out]
              }
            }
          }
        }
      }
      event "保持输出": Value Change {
        n889 = event-data() -> ()  [unwired: 1 in, 5 out]
        n890 = property on="btn_开始试验" class="Bool"("DisabledEnum"=T1."Enabled" ("禁用")) -> ()  [unwired: 2 in, 2 out]
      }
      event "btn_全选": Value Change {
        w291 = TRUE ("单选_第41路")
        n891 = event-data() -> ()  [unwired: 1 in, 5 out]
        n892 = local write "单选_第1路"(w291) -> ()
        n893 = local write "单选_第2路"(w291) -> ()
        n894 = local write "单选_第3路"(w291) -> ()
        n895 = local write "单选_第4路"(w291) -> ()
        n896 = local write "单选_第5路"(w291) -> ()
        n897 = local write "单选_第6路"(w291) -> ()
        n898 = local write "单选_第7路"(w291) -> ()
        n899 = local write "单选_第8路"(w291) -> ()
        n900 = local write "单选_第9路"(w291) -> ()
        n901 = local write "单选_第10路"(w291) -> ()
        n902 = local write "单选_第11路"(w291) -> ()
        n903 = local write "单选_第12路"(w291) -> ()
        n904 = local write "单选_第13路"(w291) -> ()
        n905 = local write "单选_第14路"(w291) -> ()
        n906 = local write "单选_第15路"(w291) -> ()
        n907 = local write "单选_第16路"(w291) -> ()
        n908 = local write "单选_第17路"(w291) -> ()
        n909 = local write "单选_第18路"(w291) -> ()
        n910 = local write "单选_第19路"(w291) -> ()
        n911 = local write "单选_第20路"(w291) -> ()
        n912 = local write "单选_第21路"(w291) -> ()
        n913 = local write "单选_第22路"(w291) -> ()
        n914 = local write "单选_第23路"(w291) -> ()
        n915 = local write "单选_第24路"(w291) -> ()
        n916 = local write "单选_第25路"(w291) -> ()
        n917 = local write "单选_第26路"(w291) -> ()
        n918 = local write "单选_第27路"(w291) -> ()
        n919 = local write "单选_第28路"(w291) -> ()
        n920 = local write "单选_第29路"(w291) -> ()
        n921 = local write "单选_第30路"(w291) -> ()
        n922 = local write "单选_第31路"(w291) -> ()
        n923 = local write "单选_第32路"(w291) -> ()
        n924 = local write "单选_第33路"(w291) -> ()
        n925 = local write "单选_第34路"(w291) -> ()
        n926 = local write "单选_第35路"(w291) -> ()
        n927 = local write "单选_第36路"(w291) -> ()
        n928 = local write "单选_第37路"(w291) -> ()
        n929 = local write "单选_第38路"(w291) -> ()
        n930 = local write "单选_第39路"(w291) -> ()
        n931 = local write "单选_第40路"(w291) -> ()
        n932 = local write "单选_第41路"(w291) -> ()
        n933 = local write "单选_第42路"(w291) -> ()
        n934 = local write "单选_第43路"(w291) -> ()
        n935 = local write "单选_第44路"(w291) -> ()
        n936 = local write "单选_第45路"(w291) -> ()
        n937 = local write "单选_第46路"(w291) -> ()
        n938 = local write "单选_第47路"(w291) -> ()
        n939 = local write "单选_第48路"(w291) -> ()
        n940 = local write "单选_第49路"(w291) -> ()
        n941 = local write "单选_第50路"(w291) -> ()
        n942 = local write "单选_第51路"(w291) -> ()
        n943 = local write "单选_第52路"(w291) -> ()
        n944 = local write "单选_第53路"(w291) -> ()
        n945 = local write "单选_第54路"(w291) -> ()
        n946 = local write "单选_第55路"(w291) -> ()
        n947 = local write "单选_第56路"(w291) -> ()
        n948 = local write "单选_第57路"(w291) -> ()
        n949 = local write "单选_第58路"(w291) -> ()
        n950 = local write "单选_第59路"(w291) -> ()
        n951 = local write "单选_第60路"(w291) -> ()
        n952 = local write "单选_第61路"(w291) -> ()
        n953 = local write "单选_第62路"(w291) -> ()
        n954 = local write "单选_第63路"(w291) -> ()
        n955 = local write "单选_第64路"(w291) -> ()
        n956 = local write "单选_第71路"(w291) -> ()
        n957 = local write "单选_第79路"(w291) -> ()
        n958 = local write "单选_第65路"(w291) -> ()
        n959 = local write "单选_第66路"(w291) -> ()
        n960 = local write "单选_第67路"(w291) -> ()
        n961 = local write "单选_第68路"(w291) -> ()
        n962 = local write "单选_第69路"(w291) -> ()
        n963 = local write "单选_第70路"(w291) -> ()
        n964 = local write "单选_第72路"(w291) -> ()
        n965 = local write "单选_第73路"(w291) -> ()
        n966 = local write "单选_第74路"(w291) -> ()
        n967 = local write "单选_第75路"(w291) -> ()
        n968 = local write "单选_第76路"(w291) -> ()
        n969 = local write "单选_第77路"(w291) -> ()
        n970 = local write "单选_第78路"(w291) -> ()
        n971 = local write "单选_第80路"(w291) -> ()
      }
      event "btn_反选": Value Change {
        n972 = event-data() -> ()  [unwired: 1 in, 5 out]
        n973 = local read "单选_第1路"() -> (w451:bool)
        n974 = local read "单选_第2路"() -> (w449:bool)
        n975 = local read "单选_第3路"() -> (w447:bool)
        n976 = local read "单选_第4路"() -> (w445:bool)
        n977 = local read "单选_第5路"() -> (w443:bool)
        n978 = local read "单选_第6路"() -> (w441:bool)
        n979 = local read "单选_第7路"() -> (w440:bool)
        n980 = local read "单选_第8路"() -> (w439:bool)
        n981 = local read "单选_第9路"() -> (w438:bool)
        n982 = local read "单选_第10路"() -> (w437:bool)
        n983 = local read "单选_第11路"() -> (w436:bool)
        n984 = local read "单选_第12路"() -> (w435:bool)
        n985 = local read "单选_第13路"() -> (w434:bool)
        n986 = local read "单选_第14路"() -> (w433:bool)
        n987 = local read "单选_第15路"() -> (w432:bool)
        n988 = local read "单选_第16路"() -> (w431:bool)
        n989 = local read "单选_第17路"() -> (w430:bool)
        n990 = local read "单选_第18路"() -> (w429:bool)
        n991 = local read "单选_第19路"() -> (w428:bool)
        n992 = local read "单选_第20路"() -> (w427:bool)
        n993 = local read "单选_第21路"() -> (w426:bool)
        n994 = local read "单选_第22路"() -> (w425:bool)
        n995 = local read "单选_第23路"() -> (w424:bool)
        n996 = local read "单选_第24路"() -> (w423:bool)
        n997 = local read "单选_第25路"() -> (w422:bool)
        n998 = local read "单选_第26路"() -> (w421:bool)
        n999 = local read "单选_第27路"() -> (w420:bool)
        n1000 = local read "单选_第28路"() -> (w419:bool)
        n1001 = local read "单选_第29路"() -> (w418:bool)
        n1002 = local read "单选_第30路"() -> (w417:bool)
        n1003 = local read "单选_第31路"() -> (w416:bool)
        n1004 = local read "单选_第32路"() -> (w415:bool)
        n1005 = local read "单选_第33路"() -> (w414:bool)
        n1006 = local read "单选_第34路"() -> (w413:bool)
        n1007 = local read "单选_第35路"() -> (w412:bool)
        n1008 = local read "单选_第36路"() -> (w411:bool)
        n1009 = local read "单选_第37路"() -> (w410:bool)
        n1010 = local read "单选_第38路"() -> (w409:bool)
        n1011 = local read "单选_第39路"() -> (w408:bool)
        n1012 = local read "单选_第40路"() -> (w407:bool)
        n1013 = Not(x=w451) -> (.not. x?=w450:bool)
        n1014 = Not(x=w449) -> (.not. x?=w448:bool)
        n1015 = Not(x=w447) -> (.not. x?=w446:bool)
        n1016 = Not(x=w445) -> (.not. x?=w444:bool)
        n1017 = Not(x=w443) -> (.not. x?=w442:bool)
        n1018 = Not(x=w441) -> (.not. x?=w406:bool)
        n1019 = Not(x=w440) -> (.not. x?=w405:bool)
        n1020 = Not(x=w439) -> (.not. x?=w404:bool)
        n1021 = Not(x=w438) -> (.not. x?=w403:bool)
        n1022 = Not(x=w437) -> (.not. x?=w402:bool)
        n1023 = Not(x=w436) -> (.not. x?=w401:bool)
        n1024 = Not(x=w435) -> (.not. x?=w400:bool)
        n1025 = Not(x=w434) -> (.not. x?=w399:bool)
        n1026 = Not(x=w433) -> (.not. x?=w398:bool)
        n1027 = Not(x=w432) -> (.not. x?=w397:bool)
        n1028 = Not(x=w431) -> (.not. x?=w396:bool)
        n1029 = Not(x=w430) -> (.not. x?=w395:bool)
        n1030 = Not(x=w429) -> (.not. x?=w394:bool)
        n1031 = Not(x=w428) -> (.not. x?=w393:bool)
        n1032 = Not(x=w427) -> (.not. x?=w392:bool)
        n1033 = Not(x=w426) -> (.not. x?=w391:bool)
        n1034 = Not(x=w425) -> (.not. x?=w390:bool)
        n1035 = Not(x=w424) -> (.not. x?=w389:bool)
        n1036 = Not(x=w423) -> (.not. x?=w388:bool)
        n1037 = Not(x=w422) -> (.not. x?=w387:bool)
        n1038 = Not(x=w421) -> (.not. x?=w386:bool)
        n1039 = Not(x=w420) -> (.not. x?=w385:bool)
        n1040 = Not(x=w419) -> (.not. x?=w384:bool)
        n1041 = Not(x=w418) -> (.not. x?=w383:bool)
        n1042 = Not(x=w417) -> (.not. x?=w382:bool)
        n1043 = Not(x=w416) -> (.not. x?=w381:bool)
        n1044 = Not(x=w415) -> (.not. x?=w380:bool)
        n1045 = Not(x=w414) -> (.not. x?=w379:bool)
        n1046 = Not(x=w413) -> (.not. x?=w378:bool)
        n1047 = Not(x=w412) -> (.not. x?=w377:bool)
        n1048 = Not(x=w411) -> (.not. x?=w376:bool)
        n1049 = Not(x=w410) -> (.not. x?=w375:bool)
        n1050 = Not(x=w409) -> (.not. x?=w374:bool)
        n1051 = Not(x=w408) -> (.not. x?=w373:bool)
        n1052 = Not(x=w407) -> (.not. x?=w372:bool)
        n1053 = local write "单选_第1路"(w450) -> ()
        n1054 = local write "单选_第2路"(w448) -> ()
        n1055 = local write "单选_第3路"(w446) -> ()
        n1056 = local write "单选_第4路"(w444) -> ()
        n1057 = local write "单选_第5路"(w442) -> ()
        n1058 = local write "单选_第6路"(w406) -> ()
        n1059 = local write "单选_第7路"(w405) -> ()
        n1060 = local write "单选_第8路"(w404) -> ()
        n1061 = local write "单选_第9路"(w403) -> ()
        n1062 = local write "单选_第10路"(w402) -> ()
        n1063 = local write "单选_第11路"(w401) -> ()
        n1064 = local write "单选_第12路"(w400) -> ()
        n1065 = local write "单选_第13路"(w399) -> ()
        n1066 = local write "单选_第14路"(w398) -> ()
        n1067 = local write "单选_第15路"(w397) -> ()
        n1068 = local write "单选_第16路"(w396) -> ()
        n1069 = local write "单选_第17路"(w395) -> ()
        n1070 = local write "单选_第18路"(w394) -> ()
        n1071 = local write "单选_第19路"(w393) -> ()
        n1072 = local write "单选_第20路"(w392) -> ()
        n1073 = local write "单选_第21路"(w391) -> ()
        n1074 = local write "单选_第22路"(w390) -> ()
        n1075 = local write "单选_第23路"(w389) -> ()
        n1076 = local write "单选_第24路"(w388) -> ()
        n1077 = local write "单选_第25路"(w387) -> ()
        n1078 = local write "单选_第26路"(w386) -> ()
        n1079 = local write "单选_第27路"(w385) -> ()
        n1080 = local write "单选_第28路"(w384) -> ()
        n1081 = local write "单选_第29路"(w383) -> ()
        n1082 = local write "单选_第30路"(w382) -> ()
        n1083 = local write "单选_第31路"(w381) -> ()
        n1084 = local write "单选_第32路"(w380) -> ()
        n1085 = local write "单选_第33路"(w379) -> ()
        n1086 = local write "单选_第34路"(w378) -> ()
        n1087 = local write "单选_第35路"(w377) -> ()
        n1088 = local write "单选_第36路"(w376) -> ()
        n1089 = local write "单选_第37路"(w375) -> ()
        n1090 = local write "单选_第38路"(w374) -> ()
        n1091 = local write "单选_第39路"(w373) -> ()
        n1092 = local write "单选_第40路"(w372) -> ()
        n1093 = local read "单选_第71路"() -> (w341:bool)
        n1094 = local read "单选_第79路"() -> (w333:bool)
        n1095 = local read "单选_第41路"() -> (w371:bool)
        n1096 = local read "单选_第42路"() -> (w370:bool)
        n1097 = local read "单选_第43路"() -> (w369:bool)
        n1098 = local read "单选_第44路"() -> (w368:bool)
        n1099 = local read "单选_第45路"() -> (w367:bool)
        n1100 = local read "单选_第46路"() -> (w366:bool)
        n1101 = local read "单选_第47路"() -> (w365:bool)
        n1102 = local read "单选_第48路"() -> (w364:bool)
        n1103 = local read "单选_第49路"() -> (w363:bool)
        n1104 = local read "单选_第50路"() -> (w362:bool)
        n1105 = local read "单选_第51路"() -> (w361:bool)
        n1106 = local read "单选_第52路"() -> (w360:bool)
        n1107 = local read "单选_第53路"() -> (w359:bool)
        n1108 = local read "单选_第54路"() -> (w358:bool)
        n1109 = local read "单选_第55路"() -> (w357:bool)
        n1110 = local read "单选_第56路"() -> (w356:bool)
        n1111 = local read "单选_第57路"() -> (w355:bool)
        n1112 = local read "单选_第58路"() -> (w354:bool)
        n1113 = local read "单选_第59路"() -> (w353:bool)
        n1114 = local read "单选_第60路"() -> (w352:bool)
        n1115 = local read "单选_第61路"() -> (w351:bool)
        n1116 = local read "单选_第62路"() -> (w350:bool)
        n1117 = local read "单选_第63路"() -> (w349:bool)
        n1118 = local read "单选_第64路"() -> (w348:bool)
        n1119 = local read "单选_第65路"() -> (w347:bool)
        n1120 = local read "单选_第66路"() -> (w346:bool)
        n1121 = local read "单选_第67路"() -> (w345:bool)
        n1122 = local read "单选_第68路"() -> (w344:bool)
        n1123 = local read "单选_第69路"() -> (w343:bool)
        n1124 = local read "单选_第70路"() -> (w342:bool)
        n1125 = local read "单选_第72路"() -> (w340:bool)
        n1126 = local read "单选_第73路"() -> (w339:bool)
        n1127 = local read "单选_第74路"() -> (w338:bool)
        n1128 = local read "单选_第75路"() -> (w337:bool)
        n1129 = local read "单选_第76路"() -> (w336:bool)
        n1130 = local read "单选_第77路"() -> (w335:bool)
        n1131 = local read "单选_第78路"() -> (w334:bool)
        n1132 = local read "单选_第80路"() -> (w332:bool)
        n1133 = Not(x=w371) -> (.not. x?=w331:bool)
        n1134 = Not(x=w370) -> (.not. x?=w330:bool)
        n1135 = Not(x=w369) -> (.not. x?=w329:bool)
        n1136 = Not(x=w368) -> (.not. x?=w328:bool)
        n1137 = Not(x=w367) -> (.not. x?=w327:bool)
        n1138 = Not(x=w366) -> (.not. x?=w326:bool)
        n1139 = Not(x=w365) -> (.not. x?=w325:bool)
        n1140 = Not(x=w364) -> (.not. x?=w324:bool)
        n1141 = Not(x=w363) -> (.not. x?=w323:bool)
        n1142 = Not(x=w362) -> (.not. x?=w322:bool)
        n1143 = Not(x=w361) -> (.not. x?=w321:bool)
        n1144 = Not(x=w360) -> (.not. x?=w320:bool)
        n1145 = Not(x=w359) -> (.not. x?=w319:bool)
        n1146 = Not(x=w358) -> (.not. x?=w318:bool)
        n1147 = Not(x=w357) -> (.not. x?=w317:bool)
        n1148 = Not(x=w356) -> (.not. x?=w316:bool)
        n1149 = Not(x=w355) -> (.not. x?=w315:bool)
        n1150 = Not(x=w354) -> (.not. x?=w314:bool)
        n1151 = Not(x=w353) -> (.not. x?=w313:bool)
        n1152 = Not(x=w352) -> (.not. x?=w312:bool)
        n1153 = Not(x=w351) -> (.not. x?=w311:bool)
        n1154 = Not(x=w350) -> (.not. x?=w310:bool)
        n1155 = Not(x=w349) -> (.not. x?=w309:bool)
        n1156 = Not(x=w348) -> (.not. x?=w308:bool)
        n1157 = Not(x=w347) -> (.not. x?=w307:bool)
        n1158 = Not(x=w346) -> (.not. x?=w306:bool)
        n1159 = Not(x=w345) -> (.not. x?=w305:bool)
        n1160 = Not(x=w344) -> (.not. x?=w304:bool)
        n1161 = Not(x=w343) -> (.not. x?=w303:bool)
        n1162 = Not(x=w342) -> (.not. x?=w302:bool)
        n1163 = Not(x=w341) -> (.not. x?=w301:bool)
        n1164 = Not(x=w340) -> (.not. x?=w300:bool)
        n1165 = Not(x=w339) -> (.not. x?=w299:bool)
        n1166 = Not(x=w338) -> (.not. x?=w298:bool)
        n1167 = Not(x=w337) -> (.not. x?=w297:bool)
        n1168 = Not(x=w336) -> (.not. x?=w296:bool)
        n1169 = Not(x=w335) -> (.not. x?=w295:bool)
        n1170 = Not(x=w334) -> (.not. x?=w294:bool)
        n1171 = Not(x=w333) -> (.not. x?=w293:bool)
        n1172 = Not(x=w332) -> (.not. x?=w292:bool)
        n1173 = local write "单选_第71路"(w301) -> ()
        n1174 = local write "单选_第79路"(w293) -> ()
        n1175 = local write "单选_第41路"(w331) -> ()
        n1176 = local write "单选_第42路"(w330) -> ()
        n1177 = local write "单选_第43路"(w329) -> ()
        n1178 = local write "单选_第44路"(w328) -> ()
        n1179 = local write "单选_第45路"(w327) -> ()
        n1180 = local write "单选_第46路"(w326) -> ()
        n1181 = local write "单选_第47路"(w325) -> ()
        n1182 = local write "单选_第48路"(w324) -> ()
        n1183 = local write "单选_第49路"(w323) -> ()
        n1184 = local write "单选_第50路"(w322) -> ()
        n1185 = local write "单选_第51路"(w321) -> ()
        n1186 = local write "单选_第52路"(w320) -> ()
        n1187 = local write "单选_第53路"(w319) -> ()
        n1188 = local write "单选_第54路"(w318) -> ()
        n1189 = local write "单选_第55路"(w317) -> ()
        n1190 = local write "单选_第56路"(w316) -> ()
        n1191 = local write "单选_第57路"(w315) -> ()
        n1192 = local write "单选_第58路"(w314) -> ()
        n1193 = local write "单选_第59路"(w313) -> ()
        n1194 = local write "单选_第60路"(w312) -> ()
        n1195 = local write "单选_第61路"(w311) -> ()
        n1196 = local write "单选_第62路"(w310) -> ()
        n1197 = local write "单选_第63路"(w309) -> ()
        n1198 = local write "单选_第64路"(w308) -> ()
        n1199 = local write "单选_第65路"(w307) -> ()
        n1200 = local write "单选_第66路"(w306) -> ()
        n1201 = local write "单选_第67路"(w305) -> ()
        n1202 = local write "单选_第68路"(w304) -> ()
        n1203 = local write "单选_第69路"(w303) -> ()
        n1204 = local write "单选_第70路"(w302) -> ()
        n1205 = local write "单选_第72路"(w300) -> ()
        n1206 = local write "单选_第73路"(w299) -> ()
        n1207 = local write "单选_第74路"(w298) -> ()
        n1208 = local write "单选_第75路"(w297) -> ()
        n1209 = local write "单选_第76路"(w296) -> ()
        n1210 = local write "单选_第77路"(w295) -> ()
        n1211 = local write "单选_第78路"(w294) -> ()
        n1212 = local write "单选_第80路"(w292) -> ()
      }
      event "btn_置1": Value Change {
        w452 = enum16{"0", "1"}."1" ("输入值_41")
        n1213 = event-data() -> ()  [unwired: 1 in, 5 out]
        n1214 = local write "输入值_1"(w452) -> ()
        n1215 = local write "输入值_2"(w452) -> ()
        n1216 = local write "输入值_3"(w452) -> ()
        n1217 = local write "输入值_4"(w452) -> ()
        n1218 = local write "输入值_5"(w452) -> ()
        n1219 = local write "输入值_6"(w452) -> ()
        n1220 = local write "输入值_7"(w452) -> ()
        n1221 = local write "输入值_8"(w452) -> ()
        n1222 = local write "输入值_9"(w452) -> ()
        n1223 = local write "输入值_10"(w452) -> ()
        n1224 = local write "输入值_11"(w452) -> ()
        n1225 = local write "输入值_12"(w452) -> ()
        n1226 = local write "输入值_13"(w452) -> ()
        n1227 = local write "输入值_14"(w452) -> ()
        n1228 = local write "输入值_15"(w452) -> ()
        n1229 = local write "输入值_16"(w452) -> ()
        n1230 = local write "输入值_17"(w452) -> ()
        n1231 = local write "输入值_18"(w452) -> ()
        n1232 = local write "输入值_19"(w452) -> ()
        n1233 = local write "输入值_20"(w452) -> ()
        n1234 = local write "输入值_21"(w452) -> ()
        n1235 = local write "输入值_22"(w452) -> ()
        n1236 = local write "输入值_23"(w452) -> ()
        n1237 = local write "输入值_24"(w452) -> ()
        n1238 = local write "输入值_25"(w452) -> ()
        n1239 = local write "输入值_26"(w452) -> ()
        n1240 = local write "输入值_27"(w452) -> ()
        n1241 = local write "输入值_28"(w452) -> ()
        n1242 = local write "输入值_29"(w452) -> ()
        n1243 = local write "输入值_30"(w452) -> ()
        n1244 = local write "输入值_31"(w452) -> ()
        n1245 = local write "输入值_32"(w452) -> ()
        n1246 = local write "输入值_33"(w452) -> ()
        n1247 = local write "输入值_34"(w452) -> ()
        n1248 = local write "输入值_35"(w452) -> ()
        n1249 = local write "输入值_36"(w452) -> ()
        n1250 = local write "输入值_37"(w452) -> ()
        n1251 = local write "输入值_38"(w452) -> ()
        n1252 = local write "输入值_39"(w452) -> ()
        n1253 = local write "输入值_40"(w452) -> ()
        n1254 = local write "输入值_41"(w452) -> ()
        n1255 = local write "输入值_42"(w452) -> ()
        n1256 = local write "输入值_43"(w452) -> ()
        n1257 = local write "输入值_44"(w452) -> ()
        n1258 = local write "输入值_45"(w452) -> ()
        n1259 = local write "输入值_46"(w452) -> ()
        n1260 = local write "输入值_47"(w452) -> ()
        n1261 = local write "输入值_48"(w452) -> ()
        n1262 = local write "输入值_49"(w452) -> ()
        n1263 = local write "输入值_50"(w452) -> ()
        n1264 = local write "输入值_51"(w452) -> ()
        n1265 = local write "输入值_52"(w452) -> ()
        n1266 = local write "输入值_53"(w452) -> ()
        n1267 = local write "输入值_54"(w452) -> ()
        n1268 = local write "输入值_55"(w452) -> ()
        n1269 = local write "输入值_56"(w452) -> ()
        n1270 = local write "输入值_57"(w452) -> ()
        n1271 = local write "输入值_58"(w452) -> ()
        n1272 = local write "输入值_59"(w452) -> ()
        n1273 = local write "输入值_60"(w452) -> ()
        n1274 = local write "输入值_61"(w452) -> ()
        n1275 = local write "输入值_62"(w452) -> ()
        n1276 = local write "输入值_63"(w452) -> ()
        n1277 = local write "输入值_64"(w452) -> ()
        n1278 = local write "输入值_65"(w452) -> ()
        n1279 = local write "输入值_66"(w452) -> ()
        n1280 = local write "输入值_67"(w452) -> ()
        n1281 = local write "输入值_68"(w452) -> ()
        n1282 = local write "输入值_69"(w452) -> ()
        n1283 = local write "输入值_70"(w452) -> ()
        n1284 = local write "输入值_71"(w452) -> ()
        n1285 = local write "输入值_72"(w452) -> ()
        n1286 = local write "输入值_73"(w452) -> ()
        n1287 = local write "输入值_74"(w452) -> ()
        n1288 = local write "输入值_75"(w452) -> ()
        n1289 = local write "输入值_76"(w452) -> ()
        n1290 = local write "输入值_77"(w452) -> ()
        n1291 = local write "输入值_78"(w452) -> ()
        n1292 = local write "输入值_79"(w452) -> ()
        n1293 = local write "输入值_80"(w452) -> ()
      }
      event "btn_置0": Value Change {
        w453 = enum16{"0", "1"}."0" ("输入值_41")
        n1294 = event-data() -> ()  [unwired: 1 in, 5 out]
        n1295 = local write "输入值_1"(w453) -> ()
        n1296 = local write "输入值_2"(w453) -> ()
        n1297 = local write "输入值_3"(w453) -> ()
        n1298 = local write "输入值_4"(w453) -> ()
        n1299 = local write "输入值_5"(w453) -> ()
        n1300 = local write "输入值_6"(w453) -> ()
        n1301 = local write "输入值_7"(w453) -> ()
        n1302 = local write "输入值_8"(w453) -> ()
        n1303 = local write "输入值_9"(w453) -> ()
        n1304 = local write "输入值_10"(w453) -> ()
        n1305 = local write "输入值_11"(w453) -> ()
        n1306 = local write "输入值_12"(w453) -> ()
        n1307 = local write "输入值_13"(w453) -> ()
        n1308 = local write "输入值_14"(w453) -> ()
        n1309 = local write "输入值_15"(w453) -> ()
        n1310 = local write "输入值_16"(w453) -> ()
        n1311 = local write "输入值_17"(w453) -> ()
        n1312 = local write "输入值_18"(w453) -> ()
        n1313 = local write "输入值_19"(w453) -> ()
        n1314 = local write "输入值_20"(w453) -> ()
        n1315 = local write "输入值_21"(w453) -> ()
        n1316 = local write "输入值_22"(w453) -> ()
        n1317 = local write "输入值_23"(w453) -> ()
        n1318 = local write "输入值_24"(w453) -> ()
        n1319 = local write "输入值_25"(w453) -> ()
        n1320 = local write "输入值_26"(w453) -> ()
        n1321 = local write "输入值_27"(w453) -> ()
        n1322 = local write "输入值_28"(w453) -> ()
        n1323 = local write "输入值_29"(w453) -> ()
        n1324 = local write "输入值_30"(w453) -> ()
        n1325 = local write "输入值_31"(w453) -> ()
        n1326 = local write "输入值_32"(w453) -> ()
        n1327 = local write "输入值_33"(w453) -> ()
        n1328 = local write "输入值_34"(w453) -> ()
        n1329 = local write "输入值_35"(w453) -> ()
        n1330 = local write "输入值_36"(w453) -> ()
        n1331 = local write "输入值_37"(w453) -> ()
        n1332 = local write "输入值_38"(w453) -> ()
        n1333 = local write "输入值_39"(w453) -> ()
        n1334 = local write "输入值_40"(w453) -> ()
        n1335 = local write "输入值_41"(w453) -> ()
        n1336 = local write "输入值_42"(w453) -> ()
        n1337 = local write "输入值_43"(w453) -> ()
        n1338 = local write "输入值_44"(w453) -> ()
        n1339 = local write "输入值_45"(w453) -> ()
        n1340 = local write "输入值_46"(w453) -> ()
        n1341 = local write "输入值_47"(w453) -> ()
        n1342 = local write "输入值_48"(w453) -> ()
        n1343 = local write "输入值_49"(w453) -> ()
        n1344 = local write "输入值_50"(w453) -> ()
        n1345 = local write "输入值_51"(w453) -> ()
        n1346 = local write "输入值_52"(w453) -> ()
        n1347 = local write "输入值_53"(w453) -> ()
        n1348 = local write "输入值_54"(w453) -> ()
        n1349 = local write "输入值_55"(w453) -> ()
        n1350 = local write "输入值_56"(w453) -> ()
        n1351 = local write "输入值_57"(w453) -> ()
        n1352 = local write "输入值_58"(w453) -> ()
        n1353 = local write "输入值_59"(w453) -> ()
        n1354 = local write "输入值_60"(w453) -> ()
        n1355 = local write "输入值_61"(w453) -> ()
        n1356 = local write "输入值_62"(w453) -> ()
        n1357 = local write "输入值_63"(w453) -> ()
        n1358 = local write "输入值_64"(w453) -> ()
        n1359 = local write "输入值_65"(w453) -> ()
        n1360 = local write "输入值_66"(w453) -> ()
        n1361 = local write "输入值_67"(w453) -> ()
        n1362 = local write "输入值_68"(w453) -> ()
        n1363 = local write "输入值_69"(w453) -> ()
        n1364 = local write "输入值_70"(w453) -> ()
        n1365 = local write "输入值_71"(w453) -> ()
        n1366 = local write "输入值_72"(w453) -> ()
        n1367 = local write "输入值_73"(w453) -> ()
        n1368 = local write "输入值_74"(w453) -> ()
        n1369 = local write "输入值_75"(w453) -> ()
        n1370 = local write "输入值_76"(w453) -> ()
        n1371 = local write "输入值_77"(w453) -> ()
        n1372 = local write "输入值_78"(w453) -> ()
        n1373 = local write "输入值_79"(w453) -> ()
        n1374 = local write "输入值_80"(w453) -> ()
      }
    }
  }
  n1375 = stacked-sequence {
    frame #0 {
      w454 = T1."Enabled" ("禁用")
      w455 = 0 ("同步_A1")
      w471 = T1."Disabled" ("禁用")
      n1376 = property on="测试结论" class="Str"("Text.TextColor"=u32 0) -> ()  [unwired: 2 in, 2 out]
      n1377 = local write "测试结论"("") -> ()
      n1378 = property on="D_IN_1" class="Tbl (严格)"("DisabledEnum"=w471) -> ()  [unwired: 2 in, 2 out]
      n1379 = property on="D_IN_2" class="Tbl (严格)"("DisabledEnum"=w471) -> ()  [unwired: 2 in, 2 out]
      n1380 = property on="D_IN_3" class="Tbl (严格)"("DisabledEnum"=w471) -> ()  [unwired: 2 in, 2 out]
      n1381 = property on="D_IN_4" class="Tbl (严格)"("DisabledEnum"=w471) -> ()  [unwired: 2 in, 2 out]
      n1382 = property on="D_IN_5" class="Tbl (严格)"("DisabledEnum"=w471) -> ()  [unwired: 2 in, 2 out]
      n1383 = property on="保持输出" class="Bool (严格)"("DisabledEnum"=w454) -> ()  [unwired: 2 in, 2 out]
      n1384 = property on="btn_开始试验" class="Bool"("DisabledEnum"=w454) -> ()  [unwired: 2 in, 2 out]
      n1385 = for {
        N: 16 -> [_]
        i -> [w475]
        n1386 = for {
          N: 4 -> [_]
          tunnel: w475 -> [w479]
          i -> [w480]
          w477 = u32 24 ("活动单元格:单元格大小:高度")
          n1387 = Bundle(w479, w480) -> (w478:cluster{i32, i32})  [unwired: 1 in]
          n1388 = property on="D_IN_1" class="Tbl (严格)"("Active Cell"=w478) -> (error out=w481:errorcluster)  [unwired: 2 in, 1 out]
          n1389 = property on="D_IN_2" class="Tbl (严格)"("Active Cell"=w478) -> ()  [unwired: 2 in, 2 out]
          n1390 = property on="D_IN_3" class="Tbl (严格)"("Active Cell"=w478) -> ()  [unwired: 2 in, 2 out]
          n1391 = property on="D_IN_4" class="Tbl (严格)"("Active Cell"=w478) -> ()  [unwired: 2 in, 2 out]
          n1392 = property on="D_IN_5" class="Tbl (严格)"("Active Cell"=w478) -> ()  [unwired: 2 in, 2 out]
          n1393 = property on="D_IN_1" class="Tbl (严格)"(error in=w481, "Height"=w477) -> ()  [unwired: 1 in, 2 out]
          n1394 = property on="D_IN_2" class="Tbl (严格)"("Height"=w477) -> ()  [unwired: 2 in, 2 out]
          n1395 = property on="D_IN_3" class="Tbl (严格)"("Height"=w477) -> ()  [unwired: 2 in, 2 out]
          n1396 = property on="D_IN_4" class="Tbl (严格)"("Height"=w477) -> ()  [unwired: 2 in, 2 out]
          n1397 = property on="D_IN_5" class="Tbl (严格)"("Height"=w477) -> ()  [unwired: 2 in, 2 out]
        }
        n1398 = Wait Until Next ms Multiple(millisecond multiple=u32 10 ("毫秒倍数")) -> ()  [unwired: 1 out]
      }
      n1399 = Initialize Array(FALSE, 5 ("维数大小"), 16 ("维数大小")) -> (w463:bool[][])
      n1400 = Initialize Array(enum16{"0", "1"}."0" ("输入值_32"), 5 ("维数大小"), 16 ("维数大小")) -> (w457:enum16{"0", "1"}[][])
      n1401 = Initialize Array("", 16 ("维数大小"), 4 ("维数大小")) -> (w465:string[][])
      n1402 = local write "关闭？"(FALSE) -> ()
      n1403 = local write "CAN端口"(u16 1 ("CAN端口")) -> ()
      n1404 = local write "数组_选择?"(w463) -> ()
      n1405 = local write "数组_输入值"(w457) -> ()
      n1406 = local write "D_IN_1"(w465) -> ()
      n1407 = local write "D_IN_2"(w465) -> ()
      n1408 = local write "D_IN_3"(w465) -> ()
      n1409 = local write "D_IN_4"(w465) -> ()
      n1410 = local write "D_IN_5"(w465) -> ()
      n1411 = local write "同步_A1"(w455) -> ()
      n1412 = local write "同步_A2"(w455) -> ()
    }
  }
  n1413 = Obtain Notifier(name (unnamed)=w4, notification data type=w4) -> (notifier out=w12:refnum<notifier>, error out=w11:errorcluster)  [unwired: 2 in, 1 out]
  n1414 = disable-structure shown="禁用" {
    frame Disabled {
      n1415 = for {
        N: 40 -> [_]
        i -> [w487]
        n1416 = Wait Until Next ms Multiple(millisecond multiple=u32 10 ("毫秒倍数")) -> ()  [unwired: 1 out]
        n1417 = Bundle(w487, "y"=-1) -> (w486:cluster{i32, "y":i32})  [unwired: 1 in]
        n1418 = property on="D_IN_1" class="Tbl (严格)"("Active Cell"=w486) -> (error out=w485:errorcluster)  [unwired: 2 in, 1 out]
        n1419 = property on="D_IN_1" class="Tbl (严格)"(error in=w485, "Cell BG Color"=u32 12369084) -> ()  [unwired: 1 in, 2 out]
      }
    }
    frame Enabled {
    }
  }
  n1420 = Obtain Notifier(name (unnamed)=w3, notification data type=w3) -> (notifier out=w2:refnum<notifier>)  [unwired: 2 in, 2 out]
  n1421 = while {
    tunnel: w12 -> [w494]
    tunnel: w11 -> [w493]
    tunnel: [w492] -> w10
    tunnel: [w491] -> w9
    tunnel: w2 -> [w489]
    stop <- w495 stop-if-true
    n1422 = Wait Until Next ms Multiple(millisecond multiple=u32 20 ("毫秒倍数")) -> ()  [unwired: 1 out]
    n1423 = Wait on Notification(notifier=w494, timeout in ms (-1)=20 ("超时毫秒(-1)"), error in (no error)=w493) -> (notifier out=w492:refnum<notifier>, notification=w499:string, error out=w491:errorcluster)  [unwired: 1 in, 1 out]
    n1424 = Equal?(x=w499, y="DInput" ("通知")) -> (x = y?=w490:bool)
    n1425 = case shown="真" w490 {
      tunnel: w489 -> [_ w500]
      frame False {
      }
      frame True {
        n1426 = stacked-sequence {
          tunnel: w500 -> [_ w509]
          frame #0 {
            n1427 = local read "保持输出"() -> (w502:bool)
            n1428 = case shown="真" w502 {
              selector: w502 -> [_ w508]
              tunnel: [w504 w507] -> w501
              frame False {
                n1429 = local read "同步_A1"() -> (w506:i32)
                n1430 = Equal?(x=w506, y=5) -> (x = y?=w504:bool)
              }
              frame True {
                n1431 = Not(x=w508) -> (.not. x?=w507:bool)
              }
            }
            n1432 = case shown="真" w501 {
              frame False {
              }
              frame True {
                n1433 = property on="保持输出" class="Bool (严格)"("DisabledEnum"=T1."Enabled" ("禁用")) -> ()  [unwired: 2 in, 2 out]
              }
            }
          }
          frame #1 {
            n1434 = local read "保持输出"() -> (w514:bool)
            n1435 = local read "数组_输入值"() -> (w511:enum16{"0", "1"}[][])
            n1436 = local read "数组_选择?"() -> (w512:bool[][])
            n1437 = local read "同步_A1"() -> (w510:i32)
            n1438 = case shown="假" w514 {
              tunnel: w510 -> [w574 _]
              tunnel: [w569 TRUE] -> w513
              frame False {
                n1439 = local read "同步_A2"() -> (w572:i32)
                n1440 = Less?(x=w572, y=5) -> (x < y?=w571:bool)
                n1441 = Equal?(x=w574, y=w572) -> (x = y?=w570:bool)
                n1442 = And(x=w570, y=w571) -> (x .and. y?=w569:bool)
              }
              frame True {
              }
            }
            n1443 = case shown="真" w513 {
              tunnel: w512 -> [_ w523]
              tunnel: w510 -> [_ w522]
              tunnel: w511 -> [_ w521]
              tunnel: w510 -> [_ w520]
              tunnel: w510 -> [_ w517]
              tunnel: w509 -> [_ w515]
              frame False {
              }
              frame True {
                n1444 = Index Array(array=w523, index (row)=w522) -> (element=w519:bool[])  [unwired: 1 in]
                n1445 = Index Array(array=w521, index (row)=w520) -> (element=w516:enum16{"0", "1"}[])  [unwired: 1 in]
                n1446 = Or Array Elements(Boolean array=w519) -> (logical OR=w518:bool)
                n1447 = case shown="真" w518 {
                  tunnel: w517 -> [_ w533]
                  tunnel: w516 -> [_ w530]
                  tunnel: w515 -> [_ w529]
                  frame False {
                    n1448 = local read "保持输出"() -> (w524:bool)
                    n1449 = case shown="假" w524 {
                      frame False {
                        n1450 = local read "同步_A2"() -> (w526:i32)
                        n1451 = local read "同步_A1"() -> (w527:i32)
                        n1452 = Increment(x=w526) -> (x+1=w525:i32)
                        n1453 = Increment(x=w527) -> (x+1=w528:i32)
                        n1454 = local write "同步_A2"(w525) -> ()
                        n1455 = local write "同步_A1"(w528) -> ()
                      }
                      frame True {
                      }
                    }
                  }
                  frame True {
                    n1456 = local read "CAN端口"() -> (w534:u16)
                    n1457 = Increment(x=w533) -> (x+1=w532:i32)
                    n1458 = call "16路数字量输入.vi"("第几组数据"=w532, "CAN端口"=w534) -> ("成功?"=w531:bool)  [unwired: 9 in]
                    n1459 = case shown="真" w531 {
                      tunnel: w530 -> [_ w541]
                      tunnel: w529 -> [_ w540]
                      frame False {
                        n1460 = local read "保持输出"() -> (w535:bool)
                        n1461 = case shown="假" w535 {
                          frame False {
                            n1462 = local read "同步_A2"() -> (w537:i32)
                            n1463 = local read "同步_A1"() -> (w538:i32)
                            n1464 = Increment(x=w537) -> (x+1=w536:i32)
                            n1465 = Increment(x=w538) -> (x+1=w539:i32)
                            n1466 = local write "同步_A2"(w536) -> ()
                            n1467 = local write "同步_A1"(w539) -> ()
                          }
                          frame True {
                          }
                        }
                      }
                      frame True {
                        n1468 = stacked-sequence {
                          tunnel: w541 -> [w547 _ _ _ _]
                          tunnel: w540 -> [_ w552 w563 _ _]
                          frame #0 {
                            n1469 = for {
                              tunnel: w547 -> [w549] mode=indexing
                              tunnel: [w548] -> w546 mode=indexing
                              n1470 = case shown="\"0\", 默认" w549 {
                                tunnel: [FALSE TRUE] -> w548
                                frame "0", Default {
                                }
                                frame "1" {
                                }
                              }
                            }
                            n1471 = Boolean Array To Number ("布尔数组至数值转换")(Boolean array=w546) -> (number=w545:u16)
                            n1472 = Split Number(x=w545) -> (hi(x)=w543:u8, lo(x)=w544:u8)
                            n1473 = Build Array(w544, w543) -> (w542:u8[])
                            n1474 = call "DO"("dataIn(U8Array)"=w542) -> ()  [unwired: 2 in, 17 out]
                          }
                          frame #1 {
                            # "修改I/O标志"
                            n1475 = local read "同步_A1"() -> (w554:i32)
                            n1476 = Equal?(x=w554, y=4) -> (x = y?=w556:bool)
                            n1477 = Equal?(x=w554, y=5) -> (x = y?=w555:bool)
                            n1478 = Or(x=w556, y=w555) -> (x .or. y?=w553:bool)
                            n1479 = case shown="真" w553 {
                              tunnel: w552 -> [_ w559]
                              frame False {
                              }
                              frame True {
                                n1480 = stacked-sequence {
                                tunnel: w559 -> [w560 _]
                                frame #0 {
                                n1481 = Send Notification "发送通知"(notification="IOCheck" ("通知"), notifier=w560) -> ()  [unwired: 1 in, 2 out]
                                }
                                frame #1 {
                                n1482 = Wait (ms)(milliseconds to wait=u32 500 ("等待时间（毫秒）")) -> ()  [unwired: 1 out]
                                }
                                }
                              }
                            }
                          }
                          frame #2 {
                            n1483 = Send Notification(notification="DICheck" ("通知"), notifier=w563) -> ()  [unwired: 1 in, 2 out]
                          }
                          frame #3 {
                            n1484 = Wait (ms)(milliseconds to wait=u32 5 ("等待时间（毫秒）")) -> ()  [unwired: 1 out]
                          }
                          frame #4 {
                            n1485 = local read "保持输出"() -> (w566:bool)
                            n1486 = case shown="假" w566 {
                              frame False {
                                n1487 = local read "同步_A1"() -> (w567:i32)
                                n1488 = Increment(x=w567) -> (x+1=w568:i32)
                                n1489 = local write "同步_A1"(w568) -> ()
                              }
                              frame True {
                              }
                            }
                          }
                        }
                      }
                    }
                  }
                }
              }
            }
          }
        }
      }
    }
    n1490 = local read "关闭？"() -> (w495:bool)
  }
  n1491 = Release Notifier(notifier=w10, error in (no error)=w9) -> ()  [unwired: 1 in, 3 out]
  n1492 = disable-structure shown="禁用" {
    frame Disabled {
      n1493 = for {
        N: 40 -> [_]
        i -> [w578]
        n1494 = for {
          N: 4 -> [_]
          tunnel: w578 -> [w586]
          i -> [w583]
          n1495 = Bundle(w586, w583) -> (w582:cluster{i32, i32})  [unwired: 1 in]
          n1496 = Quotient & Remainder(x=w586, y=2) -> (x-y*floor(x/y)=w584:i32)  [unwired: 1 out]
          n1497 = property on="D_IN_1" class="Tbl (严格)"("Active Cell"=w582) -> (error out=w580:errorcluster)  [unwired: 2 in, 1 out]
          n1498 = Equal To 0?(x=w584) -> (x = 0?=w587:bool)
          n1499 = case shown="真" w587 {
            tunnel: [u32 16448250 u32 15723488] -> w581
            frame False {
            }
            frame True {
            }
          }
          n1500 = property on="D_IN_1" class="Tbl (严格)"(error in=w580, "Cell BG Color"=w581) -> ()  [unwired: 1 in, 2 out]
        }
        n1501 = Wait Until Next ms Multiple(millisecond multiple=u32 10 ("毫秒倍数")) -> ()  [unwired: 1 out]
      }
    }
    frame Enabled {
    }
  }
  n1502 = Obtain Notifier(name (unnamed)=w1, notification data type=w1) -> (notifier out=w8:refnum<notifier>, error out=w7:errorcluster)  [unwired: 2 in, 1 out]
  n1503 = while {
    tunnel: w8 -> [w594]
    tunnel: w7 -> [w593]
    tunnel: [w592] -> w6
    tunnel: [w591] -> w5
    stop <- w596 stop-if-true
    n1504 = Wait Until Next ms Multiple(millisecond multiple=u32 20 ("毫秒倍数")) -> ()  [unwired: 1 out]
    n1505 = Wait on Notification(notifier=w594, timeout in ms (-1)=20 ("超时毫秒(-1)"), error in (no error)=w593) -> (notifier out=w592:refnum<notifier>, notification=w597:string, error out=w591:errorcluster)  [unwired: 1 in, 1 out]
    n1506 = Equal?(x=w597, y="DICheck" ("通知")) -> (x = y?=w595:bool)
    n1507 = case shown="真" w595 {
      frame False {
      }
      frame True {
        n1508 = stacked-sequence {
          frame #0 {
            w602 = u16 0
            w606 = u16 5397
            # "异常"
            # "正常"
            n1509 = Build Array(w606, u16 1285, w602) -> (w608:u16[])
            n1510 = Build Array(w606, u16 34181, u16 0 ("元素")) -> (w605:u16[])
            n1511 = Add(x=w602, y=u16 4) -> (x+y=w600:u16)
            n1512 = call "UDP接收.vi"("匹配帧信息_异常"=w605, "长度"=w600, "匹配帧信息_正常"=w608) -> ("异常_找到?"=w611:bool, "接收超时?"=w610:bool, "正常_找到?"=w603:bool)  [unwired: 5 in, 1 out]
            n1513 = case shown="真" w603 {
              frame False {
                n1514 = disable-structure shown="禁用" {
                  frame Disabled {
                    n1515 = call "显示对话框信息4"("Message"="以太网接收数据错误") -> ()  [unwired: 9 in, 2 out]
                  }
                  frame Enabled {
                  }
                }
              }
              frame True {
                n1516 = local read "保持输出"() -> (w622:bool)
                n1517 = local read "数组_输入值"() -> (w626:enum16{"0", "1"}[][])
                n1518 = local read "数组_选择?"() -> (w627:bool[][])
                n1519 = local read "CAN端口"() -> (w628:u16)
                n1520 = case shown="真" w622 {
                  tunnel: [w630 w631] -> w625
                  frame False {
                    n1521 = local read "同步_A2"() -> (w630:i32)
                  }
                  frame True {
                    n1522 = local read "同步_A1"() -> (w631:i32)
                  }
                }
                n1523 = Index Array(array=w627, index (row)=w625) -> (element=w623:bool[])  [unwired: 1 in]
                n1524 = To Unsigned Byte Integer(number=w625) -> (unsigned 8bit integer=w621:u8)
                n1525 = Index Array(array=w626, index (row)=w625) -> (element=w629:enum16{"0", "1"}[])  [unwired: 1 in]
                n1526 = Or Array Elements(Boolean array=w623) -> (logical OR=w624:bool)
                n1527 = case shown="真" w624 {
                  tunnel: w629 -> [_ w633]
                  tunnel: w621 -> [_ w637]
                  tunnel: w628 -> [_ w636]
                  tunnel: w625 -> [_ w635]
                  tunnel: w623 -> [_ w634]
                  frame False {
                  }
                  frame True {
                    n1528 = call "16路数字量输出.vi"("第几组数据"=w637, "CAN端口"=w636) -> ("成功?"=w632:bool)  [unwired: 9 in]
                    n1529 = case shown="真" w632 {
                      tunnel: w635 -> [_ w660]
                      tunnel: w634 -> [_ w652]
                      tunnel: w633 -> [_ w650]
                      frame False {
                      }
                      frame True {
                        n1530 = call "DAQNavi Assistant2"() -> ("dataOut(U8Array)"=w648:u8[])  [unwired: 2 in, 17 out]
                        n1531 = Index Array(array=w648, index #1=0 ("索引"), index #2=1 ("索引")) -> (element #1=w645:u8, element #2=w644:u8)
                        n1532 = Number To Boolean Array(number=w645) -> (Boolean array=w641:bool[])
                        n1533 = Number To Boolean Array(number=w644) -> (Boolean array=w640:bool[])
                        n1534 = local read "保持输出"() -> (w638:bool)
                        n1535 = Build Array (concatenate)(w641, w640) -> (w643:bool[])
                        n1536 = Boolean To (0,1) ("布尔值至(0,1)转换")(Boolean=w643) -> (0, 1=w642:i16[])
                        n1537 = case shown="真" w638 {
                          tunnel: [w661 w662] -> w639
                          frame False {
                            n1538 = local read "同步_A2"() -> (w661:i32)
                          }
                          frame True {
                            n1539 = local read "同步_A1"() -> (w662:i32)
                          }
                        }
                        n1540 = for {
                          tunnel: w642 -> [w668] mode=indexing
                          tunnel: w650 -> [w667] mode=indexing
                          tunnel: w652 -> [w666] mode=indexing
                          tunnel: [w663] -> w653 mode=indexing
                          tunnel: [w664] -> w654 mode=indexing
                          tunnel: [w665] -> w649 mode=indexing
                          n1541 = case shown="真" w666 {
                            tunnel: w668 -> [_ w681]
                            tunnel: w667 -> [_ w682]
                            tunnel: [cluster{u32, u32}[] [{12369084, 12369084}] ("结果") w677] -> w663
                            tunnel: ["" w679] -> w664
                            tunnel: [TRUE w678] -> w665
                            frame False {
                            }
                            frame True {
                              n1542 = Equal To 0?(x=w681) -> (x = 0?=w680:bool)
                              n1543 = To Word Integer ("转换为双字节整型")(number=w682) -> (16bit integer=w675:i16)
                              n1544 = local read "是否取反"() -> (w676:bool)
                              n1545 = Not Equal To 0?(x=w675) -> (x != 0?=w674:bool)
                              n1546 = case shown="真" w680 {
                                tunnel: ["1" "0"] -> w679
                                frame False {
                                }
                                frame True {
                                }
                              }
                              n1547 = case shown="真" w676 {
                                tunnel: w674 -> [w683 w685]
                                tunnel: [w683 w684] -> w673
                                frame False {
                                }
                                frame True {
                                n1548 = Not(x=w685) -> (.not. x?=w684:bool)
                                }
                              }
                              n1549 = Boolean To (0,1)(Boolean=w673) -> (0, 1=w672:i16)
                              n1550 = Equal?(x=w681, y=w672) -> (x = y?=w678:bool)
                              n1551 = case shown="假" w678 {
                                tunnel: [cluster{u32, u32}[] [{16711680, 16711680}] ("结果") cluster{u32, u32}[] [{6618880, 6618880}] ("结果")] -> w677
                                frame False {
                                }
                                frame True {
                                }
                              }
                            }
                          }
                        }
                        n1552 = local read "测试结论"() -> (w658:string)
                        n1553 = And Array Elements(Boolean array=w649) -> (logical AND=w651:bool)
                        n1554 = case shown="真" w651 {
                          tunnel: ["被测板卡所选择的数字量输出%d组测试故障，具体见上面试验结论！" "被测板卡所选择的数字量输出%d组测试正常！"] -> w656
                          frame False {
                          }
                          frame True {
                          }
                        }
                        n1555 = Format Into String(format string=w656, w639) -> (resulting string=w659:string)  [unwired: 2 in, 1 out]
                        n1556 = Concatenate Strings(w658, w659, "\r") -> (w655:string)
                        n1557 = local write "测试结论"(w655) -> ()
                        n1558 = case shown="4" w660 {
                          tunnel: w653 -> [w694 w747 w784 w821 w858]
                          tunnel: w654 -> [w690 w728 w765 w801 w838]
                          frame 0, Default {
                            n1559 = local read "D_IN_1"() -> (w693:string[][])
                            n1560 = Replace Array Subset(array=w693, new element=w690, index (col)=2 ("禁用的索引 (列)")) -> (w691:string[][])  [unwired: 1 in]
                            n1561 = Index Array(array=w694, index (row) #1=0 ("索引"), index (row) #2=1 ("索引"), index (row) #3=2 ("索引"), index (row) #4=3 ("索引"), index (row) #5=4 ("索引"), index (row) #6=5 ("索引"), index (row) #7=6 ("索引"), index (row) #8=7 ("索引"), index (row) #9=8 ("索引"), index (row) #10=9 ("索引"), index (row) #11=10 ("索引"), index (row) #12=11 ("索引"), index (row) #13=12 ("索引"), index (row) #14=13 ("索引"), index (row) #15=14 ("索引"), index (row) #16=15 ("索引")) -> (element #1=w710:cluster{u32, u32}[], element #2=w709:cluster{u32, u32}[], element #3=w708:cluster{u32, u32}[], element #4=w707:cluster{u32, u32}[], element #5=w706:cluster{u32, u32}[], element #6=w695:cluster{u32, u32}[], element #7=w696:cluster{u32, u32}[], element #8=w697:cluster{u32, u32}[], element #9=w698:cluster{u32, u32}[], element #10=w699:cluster{u32, u32}[], element #11=w700:cluster{u32, u32}[], element #12=w701:cluster{u32, u32}[], element #13=w702:cluster{u32, u32}[], element #14=w703:cluster{u32, u32}[], element #15=w704:cluster{u32, u32}[], element #16=w705:cluster{u32, u32}[])  [unwired: 16 in]
                            n1562 = local write "D_IN_1"(w691) -> ()
                            n1563 = property on="light_1" class="Bool (严格)"("Colors [4]"=w710) -> ()  [unwired: 2 in, 2 out]
                            n1564 = property on="light_2" class="Bool (严格)"("Colors [4]"=w709) -> ()  [unwired: 2 in, 2 out]
                            n1565 = property on="light_3" class="Bool (严格)"("Colors [4]"=w708) -> ()  [unwired: 2 in, 2 out]
                            n1566 = property on="light_4" class="Bool (严格)"("Colors [4]"=w707) -> ()  [unwired: 2 in, 2 out]
                            n1567 = property on="light_5" class="Bool (严格)"("Colors [4]"=w706) -> ()  [unwired: 2 in, 2 out]
                            n1568 = property on="light_6" class="Bool (严格)"("Colors [4]"=w695) -> ()  [unwired: 2 in, 2 out]
                            n1569 = property on="light_7" class="Bool (严格)"("Colors [4]"=w696) -> ()  [unwired: 2 in, 2 out]
                            n1570 = property on="light_8" class="Bool (严格)"("Colors [4]"=w697) -> ()  [unwired: 2 in, 2 out]
                            n1571 = property on="light_9" class="Bool (严格)"("Colors [4]"=w698) -> ()  [unwired: 2 in, 2 out]
                            n1572 = property on="light_10" class="Bool (严格)"("Colors [4]"=w699) -> ()  [unwired: 2 in, 2 out]
                            n1573 = property on="light_11" class="Bool (严格)"("Colors [4]"=w700) -> ()  [unwired: 2 in, 2 out]
                            n1574 = property on="light_12" class="Bool (严格)"("Colors [4]"=w701) -> ()  [unwired: 2 in, 2 out]
                            n1575 = property on="light_13" class="Bool (严格)"("Colors [4]"=w702) -> ()  [unwired: 2 in, 2 out]
                            n1576 = property on="light_14" class="Bool (严格)"("Colors [4]"=w703) -> ()  [unwired: 2 in, 2 out]
                            n1577 = property on="light_15" class="Bool (严格)"("Colors [4]"=w704) -> ()  [unwired: 2 in, 2 out]
                            n1578 = property on="light_16" class="Bool (严格)"("Colors [4]"=w705) -> ()  [unwired: 2 in, 2 out]
                          }
                          frame 2 {
                            n1579 = local read "D_IN_3"() -> (w729:string[][])
                            n1580 = Replace Array Subset(array=w729, new element=w728, index (col)=2 ("索引 (列)")) -> (w727:string[][])  [unwired: 1 in]
                            n1581 = Index Array(array=w747, index (row) #1=0 ("索引"), index (row) #2=1 ("索引"), index (row) #3=2 ("索引"), index (row) #4=3 ("索引"), index (row) #5=4 ("索引"), index (row) #6=5 ("索引"), index (row) #7=6 ("索引"), index (row) #8=7 ("索引"), index (row) #9=8 ("索引"), index (row) #10=9 ("索引"), index (row) #11=10 ("索引"), index (row) #12=11 ("索引"), index (row) #13=12 ("索引"), index (row) #14=13 ("索引"), index (row) #15=14 ("索引"), index (row) #16=15 ("索引")) -> (element #1=w746:cluster{u32, u32}[], element #2=w745:cluster{u32, u32}[], element #3=w744:cluster{u32, u32}[], element #4=w743:cluster{u32, u32}[], element #5=w742:cluster{u32, u32}[], element #6=w741:cluster{u32, u32}[], element #7=w740:cluster{u32, u32}[], element #8=w739:cluster{u32, u32}[], element #9=w738:cluster{u32, u32}[], element #10=w737:cluster{u32, u32}[], element #11=w736:cluster{u32, u32}[], element #12=w735:cluster{u32, u32}[], element #13=w734:cluster{u32, u32}[], element #14=w733:cluster{u32, u32}[], element #15=w732:cluster{u32, u32}[], element #16=w731:cluster{u32, u32}[])  [unwired: 16 in]
                            n1582 = local write "D_IN_3"(w727) -> ()
                            n1583 = property on="light_33" class="Bool (严格)"("Colors [4]"=w746) -> ()  [unwired: 2 in, 2 out]
                            n1584 = property on="light_34" class="Bool (严格)"("Colors [4]"=w745) -> ()  [unwired: 2 in, 2 out]
                            n1585 = property on="light_35" class="Bool (严格)"("Colors [4]"=w744) -> ()  [unwired: 2 in, 2 out]
                            n1586 = property on="light_36" class="Bool (严格)"("Colors [4]"=w743) -> ()  [unwired: 2 in, 2 out]
                            n1587 = property on="light_37" class="Bool (严格)"("Colors [4]"=w742) -> ()  [unwired: 2 in, 2 out]
                            n1588 = property on="light_38" class="Bool (严格)"("Colors [4]"=w741) -> ()  [unwired: 2 in, 2 out]
                            n1589 = property on="light_39" class="Bool (严格)"("Colors [4]"=w740) -> ()  [unwired: 2 in, 2 out]
                            n1590 = property on="light_40" class="Bool (严格)"("Colors [4]"=w739) -> ()  [unwired: 2 in, 2 out]
                            n1591 = property on="light_41" class="Bool (严格)"("Colors [4]"=w738) -> ()  [unwired: 2 in, 2 out]
                            n1592 = property on="light_42" class="Bool (严格)"("Colors [4]"=w737) -> ()  [unwired: 2 in, 2 out]
                            n1593 = property on="light_43" class="Bool (严格)"("Colors [4]"=w736) -> ()  [unwired: 2 in, 2 out]
                            n1594 = property on="light_44" class="Bool (严格)"("Colors [4]"=w735) -> ()  [unwired: 2 in, 2 out]
                            n1595 = property on="light_45" class="Bool (严格)"("Colors [4]"=w734) -> ()  [unwired: 2 in, 2 out]
                            n1596 = property on="light_46" class="Bool (严格)"("Colors [4]"=w733) -> ()  [unwired: 2 in, 2 out]
                            n1597 = property on="light_47" class="Bool (严格)"("Colors [4]"=w732) -> ()  [unwired: 2 in, 2 out]
                            n1598 = property on="light_48" class="Bool (严格)"("Colors [4]"=w731) -> ()  [unwired: 2 in, 2 out]
                          }
                          frame 3 {
                            n1599 = local read "D_IN_4"() -> (w766:string[][])
                            n1600 = Replace Array Subset(array=w766, new element=w765, index (col)=2 ("索引 (列)")) -> (w764:string[][])  [unwired: 1 in]
                            n1601 = Index Array(array=w784, index (row) #1=0 ("索引"), index (row) #2=1 ("索引"), index (row) #3=2 ("索引"), index (row) #4=3 ("索引"), index (row) #5=4 ("索引"), index (row) #6=5 ("索引"), index (row) #7=6 ("索引"), index (row) #8=7 ("索引"), index (row) #9=8 ("索引"), index (row) #10=9 ("索引"), index (row) #11=10 ("索引"), index (row) #12=11 ("索引"), index (row) #13=12 ("索引"), index (row) #14=13 ("索引"), index (row) #15=14 ("索引"), index (row) #16=15 ("索引")) -> (element #1=w783:cluster{u32, u32}[], element #2=w782:cluster{u32, u32}[], element #3=w781:cluster{u32, u32}[], element #4=w780:cluster{u32, u32}[], element #5=w779:cluster{u32, u32}[], element #6=w778:cluster{u32, u32}[], element #7=w777:cluster{u32, u32}[], element #8=w776:cluster{u32, u32}[], element #9=w775:cluster{u32, u32}[], element #10=w774:cluster{u32, u32}[], element #11=w773:cluster{u32, u32}[], element #12=w772:cluster{u32, u32}[], element #13=w771:cluster{u32, u32}[], element #14=w770:cluster{u32, u32}[], element #15=w769:cluster{u32, u32}[], element #16=w768:cluster{u32, u32}[])  [unwired: 16 in]
                            n1602 = local write "D_IN_4"(w764) -> ()
                            n1603 = property on="light_49" class="Bool (严格)"("Colors [4]"=w783) -> ()  [unwired: 2 in, 2 out]
                            n1604 = property on="light_50" class="Bool (严格)"("Colors [4]"=w782) -> ()  [unwired: 2 in, 2 out]
                            n1605 = property on="light_51" class="Bool (严格)"("Colors [4]"=w781) -> ()  [unwired: 2 in, 2 out]
                            n1606 = property on="light_52" class="Bool (严格)"("Colors [4]"=w780) -> ()  [unwired: 2 in, 2 out]
                            n1607 = property on="light_53" class="Bool (严格)"("Colors [4]"=w779) -> ()  [unwired: 2 in, 2 out]
                            n1608 = property on="light_54" class="Bool (严格)"("Colors [4]"=w778) -> ()  [unwired: 2 in, 2 out]
                            n1609 = property on="light_55" class="Bool (严格)"("Colors [4]"=w777) -> ()  [unwired: 2 in, 2 out]
                            n1610 = property on="light_56" class="Bool (严格)"("Colors [4]"=w776) -> ()  [unwired: 2 in, 2 out]
                            n1611 = property on="light_57" class="Bool (严格)"("Colors [4]"=w775) -> ()  [unwired: 2 in, 2 out]
                            n1612 = property on="light_58" class="Bool (严格)"("Colors [4]"=w774) -> ()  [unwired: 2 in, 2 out]
                            n1613 = property on="light_59" class="Bool (严格)"("Colors [4]"=w773) -> ()  [unwired: 2 in, 2 out]
                            n1614 = property on="light_60" class="Bool (严格)"("Colors [4]"=w772) -> ()  [unwired: 2 in, 2 out]
                            n1615 = property on="light_61" class="Bool (严格)"("Colors [4]"=w771) -> ()  [unwired: 2 in, 2 out]
                            n1616 = property on="light_62" class="Bool (严格)"("Colors [4]"=w770) -> ()  [unwired: 2 in, 2 out]
                            n1617 = property on="light_63" class="Bool (严格)"("Colors [4]"=w769) -> ()  [unwired: 2 in, 2 out]
                            n1618 = property on="light_64" class="Bool (严格)"("Colors [4]"=w768) -> ()  [unwired: 2 in, 2 out]
                          }
                          frame 4 {
                            n1619 = local read "D_IN_5"() -> (w803:string[][])
                            n1620 = Replace Array Subset(array=w803, new element=w801, index (col)=2 ("索引 (列)")) -> (w802:string[][])  [unwired: 1 in]
                            n1621 = Index Array(array=w821, index (row) #1=0 ("索引"), index (row) #2=1 ("索引"), index (row) #3=2 ("索引"), index (row) #4=3 ("索引"), index (row) #5=4 ("索引"), index (row) #6=5 ("索引"), index (row) #7=6 ("索引"), index (row) #8=7 ("索引"), index (row) #9=8 ("索引"), index (row) #10=9 ("索引"), index (row) #11=10 ("索引"), index (row) #12=11 ("索引"), index (row) #13=12 ("索引"), index (row) #14=13 ("索引"), index (row) #15=14 ("索引"), index (row) #16=15 ("索引")) -> (element #1=w820:cluster{u32, u32}[], element #2=w819:cluster{u32, u32}[], element #3=w818:cluster{u32, u32}[], element #4=w817:cluster{u32, u32}[], element #5=w816:cluster{u32, u32}[], element #6=w815:cluster{u32, u32}[], element #7=w814:cluster{u32, u32}[], element #8=w813:cluster{u32, u32}[], element #9=w812:cluster{u32, u32}[], element #10=w811:cluster{u32, u32}[], element #11=w810:cluster{u32, u32}[], element #12=w809:cluster{u32, u32}[], element #13=w808:cluster{u32, u32}[], element #14=w807:cluster{u32, u32}[], element #15=w806:cluster{u32, u32}[], element #16=w805:cluster{u32, u32}[])  [unwired: 16 in]
                            n1622 = local write "D_IN_5"(w802) -> ()
                            n1623 = property on="light_65" class="Bool (严格)"("Colors [4]"=w820) -> ()  [unwired: 2 in, 2 out]
                            n1624 = property on="light_66" class="Bool (严格)"("Colors [4]"=w819) -> ()  [unwired: 2 in, 2 out]
                            n1625 = property on="light_67" class="Bool (严格)"("Colors [4]"=w818) -> ()  [unwired: 2 in, 2 out]
                            n1626 = property on="light_68" class="Bool (严格)"("Colors [4]"=w817) -> ()  [unwired: 2 in, 2 out]
                            n1627 = property on="light_69" class="Bool (严格)"("Colors [4]"=w816) -> ()  [unwired: 2 in, 2 out]
                            n1628 = property on="light_70" class="Bool (严格)"("Colors [4]"=w815) -> ()  [unwired: 2 in, 2 out]
                            n1629 = property on="light_71" class="Bool (严格)"("Colors [4]"=w814) -> ()  [unwired: 2 in, 2 out]
                            n1630 = property on="light_72" class="Bool (严格)"("Colors [4]"=w813) -> ()  [unwired: 2 in, 2 out]
                            n1631 = property on="light_73" class="Bool (严格)"("Colors [4]"=w812) -> ()  [unwired: 2 in, 2 out]
                            n1632 = property on="light_74" class="Bool (严格)"("Colors [4]"=w811) -> ()  [unwired: 2 in, 2 out]
                            n1633 = property on="light_75" class="Bool (严格)"("Colors [4]"=w810) -> ()  [unwired: 2 in, 2 out]
                            n1634 = property on="light_76" class="Bool (严格)"("Colors [4]"=w809) -> ()  [unwired: 2 in, 2 out]
                            n1635 = property on="light_77" class="Bool (严格)"("Colors [4]"=w808) -> ()  [unwired: 2 in, 2 out]
                            n1636 = property on="light_78" class="Bool (严格)"("Colors [4]"=w807) -> ()  [unwired: 2 in, 2 out]
                            n1637 = property on="light_79" class="Bool (严格)"("Colors [4]"=w806) -> ()  [unwired: 2 in, 2 out]
                            n1638 = property on="light_80" class="Bool (严格)"("Colors [4]"=w805) -> ()  [unwired: 2 in, 2 out]
                          }
                          frame 1 {
                            n1639 = local read "D_IN_2"() -> (w840:string[][])
                            n1640 = Replace Array Subset(array=w840, new element=w838, index (col)=2 ("索引 (列)")) -> (w839:string[][])  [unwired: 1 in]
                            n1641 = Index Array(array=w858, index (row) #1=0 ("索引"), index (row) #2=1 ("索引"), index (row) #3=2 ("索引"), index (row) #4=3 ("索引"), index (row) #5=4 ("索引"), index (row) #6=5 ("索引"), index (row) #7=6 ("索引"), index (row) #8=7 ("索引"), index (row) #9=8 ("索引"), index (row) #10=9 ("索引"), index (row) #11=10 ("索引"), index (row) #12=11 ("索引"), index (row) #13=12 ("索引"), index (row) #14=13 ("索引"), index (row) #15=14 ("索引"), index (row) #16=15 ("索引")) -> (element #1=w857:cluster{u32, u32}[], element #2=w856:cluster{u32, u32}[], element #3=w855:cluster{u32, u32}[], element #4=w854:cluster{u32, u32}[], element #5=w853:cluster{u32, u32}[], element #6=w852:cluster{u32, u32}[], element #7=w851:cluster{u32, u32}[], element #8=w850:cluster{u32, u32}[], element #9=w849:cluster{u32, u32}[], element #10=w848:cluster{u32, u32}[], element #11=w847:cluster{u32, u32}[], element #12=w846:cluster{u32, u32}[], element #13=w845:cluster{u32, u32}[], element #14=w844:cluster{u32, u32}[], element #15=w843:cluster{u32, u32}[], element #16=w842:cluster{u32, u32}[])  [unwired: 16 in]
                            n1642 = local write "D_IN_2"(w839) -> ()
                            n1643 = property on="light_17" class="Bool (严格)"("Colors [4]"=w857) -> ()  [unwired: 2 in, 2 out]
                            n1644 = property on="light_18" class="Bool (严格)"("Colors [4]"=w856) -> ()  [unwired: 2 in, 2 out]
                            n1645 = property on="light_19" class="Bool (严格)"("Colors [4]"=w855) -> ()  [unwired: 2 in, 2 out]
                            n1646 = property on="light_20" class="Bool (严格)"("Colors [4]"=w854) -> ()  [unwired: 2 in, 2 out]
                            n1647 = property on="light_21" class="Bool (严格)"("Colors [4]"=w853) -> ()  [unwired: 2 in, 2 out]
                            n1648 = property on="light_22" class="Bool (严格)"("Colors [4]"=w852) -> ()  [unwired: 2 in, 2 out]
                            n1649 = property on="light_23" class="Bool (严格)"("Colors [4]"=w851) -> ()  [unwired: 2 in, 2 out]
                            n1650 = property on="light_24" class="Bool (严格)"("Colors [4]"=w850) -> ()  [unwired: 2 in, 2 out]
                            n1651 = property on="light_25" class="Bool (严格)"("Colors [4]"=w849) -> ()  [unwired: 2 in, 2 out]
                            n1652 = property on="light_26" class="Bool (严格)"("Colors [4]"=w848) -> ()  [unwired: 2 in, 2 out]
                            n1653 = property on="light_27" class="Bool (严格)"("Colors [4]"=w847) -> ()  [unwired: 2 in, 2 out]
                            n1654 = property on="light_28" class="Bool (严格)"("Colors [4]"=w846) -> ()  [unwired: 2 in, 2 out]
                            n1655 = property on="light_29" class="Bool (严格)"("Colors [4]"=w845) -> ()  [unwired: 2 in, 2 out]
                            n1656 = property on="light_30" class="Bool (严格)"("Colors [4]"=w844) -> ()  [unwired: 2 in, 2 out]
                            n1657 = property on="light_31" class="Bool (严格)"("Colors [4]"=w843) -> ()  [unwired: 2 in, 2 out]
                            n1658 = property on="light_32" class="Bool (严格)"("Colors [4]"=w842) -> ()  [unwired: 2 in, 2 out]
                          }
                        }
                      }
                    }
                  }
                }
              }
            }
            n1659 = case shown="真" w610 {
              frame False {
              }
              frame True {
                n1660 = call "显示对话框信息3"("Message"="数字量输出数值修改超时") -> ("结束"=w612:bool)  [unwired: 9 in, 1 out]
                n1661 = case shown="真" w612 {
                  frame False {
                  }
                  frame True {
                    n1662 = local write "同步_A1"(5 ("同步_A1")) -> ()
                    n1663 = local write "保持输出"(FALSE ("保持输出")) -> ()
                  }
                }
              }
            }
            n1664 = case shown="真" w611 {
              frame False {
              }
              frame True {
                n1665 = call "显示对话框信息2"("Message"="数字量输出数值修改失败") -> ("结束"=w616:bool)  [unwired: 9 in, 1 out]
                n1666 = case shown="真" w616 {
                  frame False {
                  }
                  frame True {
                    n1667 = local write "同步_A1"(5 ("同步_A1")) -> ()
                    n1668 = local write "保持输出"(FALSE ("保持输出")) -> ()
                  }
                }
              }
            }
          }
          frame #1 {
            n1669 = local read "保持输出"() -> (w877:bool)
            n1670 = case shown="假" w877 {
              frame False {
                n1671 = local read "同步_A2"() -> (w878:i32)
                n1672 = Increment(x=w878) -> (x+1=w879:i32)
                n1673 = local write "同步_A2"(w879) -> ()
              }
              frame True {
              }
            }
          }
        }
      }
    }
    n1674 = local read "关闭？"() -> (w596:bool)
  }
  n1675 = Release Notifier(notifier=w6, error in (no error)=w5) -> ()  [unwired: 1 in, 3 out]
